vi "Dashboard Main.vi"() -> ()   [LabVIEW 2020]
uses:
  <vilib>/Utility/miscctls.llb/LVRectTypeDef.ctl
  <vilib>/event_ctls.llb/eventvkey.ctl
  <vilib>/Rock Robotics/WPI/DriverStation/WPI_DriverStationAllianceInfo.ctl
  b1c29fd4-b69e-4c47-bd92-218700034153.vi
  efc637a3-a7e0-4d6a-acb3-aee6468bd1cb.vi
  b2059994-562a-4507-8104-e4c00853bec9.vi
  7fc597ec-ac8e-4325-b133-71466b1fbbcb.vi
  9cac3b8b-4a3f-4d18-bfb1-3aae72e664f2.vi
  a7551b2b-ce58-4830-98e7-c5cf61f6feb4.vi
  cd51690b-7cbe-44fb-a5f0-3232adb0ed53.vi
  a4e8d5d1-2ec3-4e81-be0b-60391cc68073.vi
  1b78be80-bab2-445d-a3e8-82f142a16380.vi
  9e807339-2903-4f51-8fcc-64b6a9381567.vi
  e75f20ac-3dfa-4544-8614-4803d6d17fbb.vi
  273c17a0-a238-4f2a-a55a-7e29d73850ff.vi
  87bdd142-1820-4e26-8582-f713a5f3da40.vi
  b8451b18-7b16-4e07-a196-a1bebf8ce026.vi
  5d307e9f-edd0-4132-a387-09c5916d43b1.vi
  0137daef-9682-45ba-80b9-2d4fda8852b8.vi
  f6a63fab-964b-4051-8314-d4414a0a258c.vi
  90e0fe9d-42b1-4a72-a6c8-4b9d9b3a5a2a.vi
  f15e925d-3118-43e3-bf67-a1272bbf81dd.vi
  394886aa-4cdd-4740-8681-89e3e438764a.vi
  77a42c1f-99bf-4bb6-8218-45b49017f7dc.vi
  5abae45b-ab2b-4816-ba0c-2a0b218f6531.vi
  31f70c1d-3051-4c77-9544-a691198ba614.vi
  f63f5451-5db6-487e-bc86-5cb81e92b132.vi
  81d0db6a-d68a-45c3-b3b1-458879412541.vi
  c235c188-eb56-46fb-93d3-e8acf396af31.vi
  115ba94a-0b26-47fa-ae73-5ec5bd9e502a.vi
  2422668c-951b-48e5-9bda-0f59c56d9c0d.vi
  7776664e-4af7-4b3d-b288-2266642a045e.vi
  6004ed5d-dfc4-4dad-95c1-8e371ea2b9cd.vi
  321ce103-7778-4bb1-9ecc-75a76fef05e9.vi
  d30e88cc-5e2b-4867-b271-53fc6d5cd4d7.vi
  fde90579-e212-4b8a-8145-a17c3e40bcbd.vi
  6c63589b-432e-4f9c-bacb-2063ed7bd576.vi
  b7dcf304-99f6-4f78-9d14-19aa8d9ea562.vi
  e8b3bb93-ba91-445b-94c6-9e998421f827.vi
  0480a820-69ef-45e6-a9f4-d7ff60c89e45.vi
  1c99237e-ea3d-4ecf-b7c2-61034db3ecd2.vi
  0a8fe2ab-d060-4915-a9b5-d8978247e2b6.vi
  bcb69d65-de6b-4edb-ab22-bddb8ff6e42b.vi
  9102154a-bccf-464c-9607-78527809ea41.vi
  bef7421f-6b7f-4c9f-a030-6027c2463e15.vi
  88deb554-0c34-4998-a7e4-ba2d14003654.vi
  b1c29fd4-b69e-4c47-bd92-218700034153.vi/77c742ae-e671-49bb-a825-a6e8cebc9f63.vi
  b2059994-562a-4507-8104-e4c00853bec9.vi/77c742ae-e671-49bb-a825-a6e8cebc9f63.vi
  9cac3b8b-4a3f-4d18-bfb1-3aae72e664f2.vi/77c742ae-e671-49bb-a825-a6e8cebc9f63.vi
  a7551b2b-ce58-4830-98e7-c5cf61f6feb4.vi/77c742ae-e671-49bb-a825-a6e8cebc9f63.vi
  cd51690b-7cbe-44fb-a5f0-3232adb0ed53.vi/77c742ae-e671-49bb-a825-a6e8cebc9f63.vi
  a4e8d5d1-2ec3-4e81-be0b-60391cc68073.vi/77c742ae-e671-49bb-a825-a6e8cebc9f63.vi
  1b78be80-bab2-445d-a3e8-82f142a16380.vi/77c742ae-e671-49bb-a825-a6e8cebc9f63.vi
  9e807339-2903-4f51-8fcc-64b6a9381567.vi/77c742ae-e671-49bb-a825-a6e8cebc9f63.vi
  e75f20ac-3dfa-4544-8614-4803d6d17fbb.vi/77c742ae-e671-49bb-a825-a6e8cebc9f63.vi
  0137daef-9682-45ba-80b9-2d4fda8852b8.vi/77c742ae-e671-49bb-a825-a6e8cebc9f63.vi
  f6a63fab-964b-4051-8314-d4414a0a258c.vi/77c742ae-e671-49bb-a825-a6e8cebc9f63.vi
  90e0fe9d-42b1-4a72-a6c8-4b9d9b3a5a2a.vi/77c742ae-e671-49bb-a825-a6e8cebc9f63.vi
  f15e925d-3118-43e3-bf67-a1272bbf81dd.vi/77c742ae-e671-49bb-a825-a6e8cebc9f63.vi
  394886aa-4cdd-4740-8681-89e3e438764a.vi/77c742ae-e671-49bb-a825-a6e8cebc9f63.vi
  77a42c1f-99bf-4bb6-8218-45b49017f7dc.vi/77c742ae-e671-49bb-a825-a6e8cebc9f63.vi
  5abae45b-ab2b-4816-ba0c-2a0b218f6531.vi/77c742ae-e671-49bb-a825-a6e8cebc9f63.vi
  31f70c1d-3051-4c77-9544-a691198ba614.vi/77c742ae-e671-49bb-a825-a6e8cebc9f63.vi
  f63f5451-5db6-487e-bc86-5cb81e92b132.vi/77c742ae-e671-49bb-a825-a6e8cebc9f63.vi
  81d0db6a-d68a-45c3-b3b1-458879412541.vi/77c742ae-e671-49bb-a825-a6e8cebc9f63.vi
  c235c188-eb56-46fb-93d3-e8acf396af31.vi/77c742ae-e671-49bb-a825-a6e8cebc9f63.vi
  115ba94a-0b26-47fa-ae73-5ec5bd9e502a.vi/77c742ae-e671-49bb-a825-a6e8cebc9f63.vi
  2422668c-951b-48e5-9bda-0f59c56d9c0d.vi/77c742ae-e671-49bb-a825-a6e8cebc9f63.vi
  7776664e-4af7-4b3d-b288-2266642a045e.vi/77c742ae-e671-49bb-a825-a6e8cebc9f63.vi
  6004ed5d-dfc4-4dad-95c1-8e371ea2b9cd.vi/77c742ae-e671-49bb-a825-a6e8cebc9f63.vi
  321ce103-7778-4bb1-9ecc-75a76fef05e9.vi/77c742ae-e671-49bb-a825-a6e8cebc9f63.vi
  d30e88cc-5e2b-4867-b271-53fc6d5cd4d7.vi/77c742ae-e671-49bb-a825-a6e8cebc9f63.vi
  fde90579-e212-4b8a-8145-a17c3e40bcbd.vi/77c742ae-e671-49bb-a825-a6e8cebc9f63.vi
  6c63589b-432e-4f9c-bacb-2063ed7bd576.vi/77c742ae-e671-49bb-a825-a6e8cebc9f63.vi
  b7dcf304-99f6-4f78-9d14-19aa8d9ea562.vi/77c742ae-e671-49bb-a825-a6e8cebc9f63.vi
  e8b3bb93-ba91-445b-94c6-9e998421f827.vi/77c742ae-e671-49bb-a825-a6e8cebc9f63.vi
  0480a820-69ef-45e6-a9f4-d7ff60c89e45.vi/77c742ae-e671-49bb-a825-a6e8cebc9f63.vi
  1c99237e-ea3d-4ecf-b7c2-61034db3ecd2.vi/77c742ae-e671-49bb-a825-a6e8cebc9f63.vi
  0a8fe2ab-d060-4915-a9b5-d8978247e2b6.vi/77c742ae-e671-49bb-a825-a6e8cebc9f63.vi
  bcb69d65-de6b-4edb-ab22-bddb8ff6e42b.vi/77c742ae-e671-49bb-a825-a6e8cebc9f63.vi
  9102154a-bccf-464c-9607-78527809ea41.vi/77c742ae-e671-49bb-a825-a6e8cebc9f63.vi
  bef7421f-6b7f-4c9f-a030-6027c2463e15.vi/77c742ae-e671-49bb-a825-a6e8cebc9f63.vi
  88deb554-0c34-4998-a7e4-ba2d14003654.vi/77c742ae-e671-49bb-a825-a6e8cebc9f63.vi
  <vilib>/Utility/xml.llb/Read From XML File(array).vi
  <vilib>/Utility/xml.llb/Write to XML File(string).vi
  <vilib>/Rock Robotics/Network Tables/NT Read Number.vi
  <vilib>/Rock Robotics/Network Tables/NT Read Boolean.vi
  GlobalDashboard.vi
  <vilib>/Rock Robotics/Network Tables/NT Read String.vi
  <vilib>/Rock Robotics/Network Tables/NT Write Number.vi
  <vilib>/Rock Robotics/Network Tables/NT Read Numeric Array.vi
  <vilib>/Rock Robotics/Network Tables/NT Write Boolean.vi
  <vilib>/Rock Robotics/Network Tables/NT Read String Array.vi
  <vilib>/Rock Robotics/Network Tables/NT Write String.vi
  <vilib>/Rock Robotics/Network Tables/NT Write Numeric Array.vi
  <vilib>/Rock Robotics/Network Tables/NT Write Integer Array.vi
  <vilib>/Rock Robotics/Network Tables/NT Write Boolean Array.vi
  <vilib>/Rock Robotics/Network Tables/NT Write String Array.vi
  <vilib>/vision/NI_Vision_Development_Module.lvlib
panel:
  in  "TCP":refnum<k5>
  in  "Dashboard Tab":T1(tab)=enum."Setup/Auto"
  in  "CheckList":i32(listbox)
  out "TOF_Range":dbl format="%.1f"
  in  "Apply_Grid_Calibration":bool
  out "Current_Red_Calibration":dbl format="%.1f"
  in  "New_Red_Calibration":dbl format="%.1f"
  out "Heading_to_Target":dbl format="%.1f"
  out "Distance_to_Target":dbl format="%.1f"
  out "Robot_P":dbl format="%.1f"
  in  "Enable_Streaming_GUI":bool=TRUE
  out "Robot_Profile_GUI":string
  out "Auto_Playbook_GUI":string
  in  "Select Driver Profile":u16(ring) items=["N/A"]
  in  "Camera Name":string(combo)="limelight"
  in  "Camera Settings":T2={"Frame Rate"=20, "Compression"=60, "Size"=1, "DB Camera Config"=FALSE} {"Size" items=["640x480", "320x240", "160x120"]}
  in  "Select Autonomous Play":u16(ring) items=["N/A"]
  out "Master_Caution_GUI_0":bool caption="Mode_Butterfly"
  out "Robot_is_Autonomous_GUI_0":bool caption="Mode_Butterfly"
  out "Robot_Code_Version_GUI":string
  out "Auto_Suffix_GUI":string
  in  "Refresh_Auto_Play_List_GUI":bool
  in  "Auto_Delay_GUI":dbl format="%.1f"
  in  "Manual_Start_X":dbl min=0.0 max=700.0 format="%.1f"
  out "Robot_X":dbl format="%.1f"
  out "Robot_Y":dbl format="%.1f"
  in  "Manual_Start_Y":dbl min=0.0 max=400.0 format="%.1f"
  out "Robot_H_GUI":dbl format="%.1f"
  in  "Manual_Start_H":dbl min=0.0 max=360.0 format="%.1f"
  in  "Field Map":u16(ring) items=["N/A"]
  in  "Push_Robot_Start_GUI":bool
  in  "Export_Robot_Pose":bool
  in  "Clear_Robot_Pose_Display":bool
  in  "Dock_Dashboard":bool
  in  "Force_Human_Control_GUI":bool
  in  "Auto_Test_Mode_GUI":bool
  in  "Disable_Fusion_While_Autonomous":bool
  in  "Disable_Fusion_While_Disabled":bool=TRUE
  out "Robot Pose 1":cluster{dbl[], dbl[]}[](graph)
  in  "New_Blue_Calibration":dbl format="%.1f"
  out "Current_Blue_Calibration":dbl format="%.1f"
  out "Help Graphic":T3(plugin-control)
  out "LL_Ret_Left":bool
  out "LL_Ret_Right":bool
  out "WA_Ret_Right":bool
  out "WA_Ret_Left":bool
  out "Swerve_Drive_Fault":bool
  out "Robot Pose 2":cluster{dbl[], dbl[]}[](graph)
  out "Vision_Fault_GUI":bool
  out "Pressure_Leak_GUI":bool
  in  "Master_Safety_Override_1":bool
  in  "Manipulator_Help":bool
  in  "Driver_Help":bool
  out "No_Secondary_Camera":bool
  out "Swerve_Shifter_Failure":bool
  out "Electrical_Fault_GUI":bool
  out "Diverting_Power_GUI":bool
  out "CAN_Bus_Fault_GUI":bool
  out "IMU_Failure_GUI":bool
  out "Robot_is_Autonomous_GUI_1":bool caption="Mode_Butterfly"
  out "LL_Valid":bool caption="Mode_Butterfly"
  out "Auto_Error_GUI":bool
  in  "Clear_Errors_GUI":bool
  out "Swerve_Azimuth_Fault":bool
  out "Pressure_Transducer_GUI":dbl(slide) scale=0.0..115.0
  out "Pressure_Vent_GUI":bool
  out "Swerve_Overheating":bool
  out "Compressor_On_GUI":bool
  in  "Right":bool
  in  "Reticule":T4(ring)
  in  "Save":bool
  in  "Up":bool
  in  "Down":bool
  in  "Left":bool
  out "Master_Caution_GUI_1":bool caption="Mode_Butterfly"
  out "Battery_Critical_GUI":bool
  out "Battery_Voltage_GUI":dbl(slide) scale=11.0..13.0
  out "Field_Oriented_GUI":bool caption="Mode_Butterfly"
  out "Slow_Loop":bool
  out "Combined Camera Feed":T3(plugin-control)
  in  "Camera_Override_GUI":bool
  in  "Field_Oriented_Override_GUI":bool
  out "Pointed_at_Target":bool caption="Mode_Butterfly"
  in  "Auto_Targeting_Override":bool
  out "Using_Auto_Targeting":bool caption="Mode_Butterfly"
  out "Solenoid 4 Numeric Display":dbl
  out "Sensor 4 Boolean Display":bool
  out "Solenoid 3 Numeric Display":dbl
  out "Sensor 3 Boolean Display":bool
  out "Solenoid 2 Numeric Display":dbl
  out "Sensor 2 Boolean Display":bool
  out "Solenoid 1 Numeric Display":dbl
  out "Sensor 1 Boolean Display":bool
  in  "Motor 8 Button Selector":T5(ring)
  in  "Motor 8 Amplitude":dbl(slide) caption="Slide" min=-1.0 max=1.0 step=0.1 scale=-1.0..1.0
  in  "Motor 7 Button Selector":T5(ring)
  in  "Motor 7 Amplitude":dbl(slide) caption="Slide" min=-1.0 max=1.0 step=0.1 scale=-1.0..1.0
  in  "Motor 6 Button Selector":T5(ring)
  in  "Motor 6 Amplitude":dbl(slide) caption="Slide" min=-1.0 max=1.0 step=0.1 scale=-1.0..1.0
  in  "Motor 5 Button Selector":T5(ring)
  in  "Motor 5 Amplitude":dbl(slide) caption="Slide" min=-1.0 max=1.0 step=0.1 scale=-1.0..1.0
  in  "Motor 4 Button Selector":T5(ring)
  in  "Motor 4 Amplitude":dbl(slide) caption="Slide" min=-1.0 max=1.0 step=0.1 scale=-1.0..1.0
  in  "Motor 3 Button Selector":T5(ring)
  in  "Motor 3 Amplitude":dbl(slide) caption="Slide" min=-1.0 max=1.0 step=0.1 scale=-1.0..1.0
  in  "Motor 2 Button Selector":T5(ring)
  in  "Motor 2 Amplitude":dbl(slide) caption="Slide" min=-1.0 max=1.0 step=0.1 scale=-1.0..1.0
  in  "Solenoid 4 Toggle":bool
  in  "Solenoid 4 Selector":T6(ring)
  in  "Solenoid 3 Toggle":bool
  in  "Solenoid 3 Selector":T6(ring)
  in  "Solenoid 2 Toggle":bool
  in  "Solenoid 2 Selector":T6(ring)
  in  "Solenoid 1 Toggle":bool
  in  "Solenoid 1 Selector":T6(ring)
  in  "Motor 1 Button Selector":T5(ring)
  in  "Motor 1 Amplitude":dbl(slide) caption="Slide" min=-1.0 max=1.0 step=0.1 scale=-1.0..1.0
  out "Swerve_Output_Loop_Time_GU":u32
  out "Swerve_3_Drive_Velocity":dbl format="%.1f"
  out "Swerve_3_Azimuth_Position":dbl format="%.1f"
  out "Swerve_3_Drive_Temperature":dbl
  out "Swerve_0_Drive_Temperature":dbl
  out "Camera Perf":string
  out "Control_Loop_Time_GUI":u32
  in  "Calibrate_Wheels_GUI":bool
  in  "Home_Wheels_GUI":bool
  out "Swerve_0_Azimuth_Position":dbl format="%.1f"
  out "Swerve_0_Drive_Velocity":dbl format="%.1f"
  out "Swerve_1_Drive_Velocity":dbl format="%.1f"
  out "Swerve_1_Azimuth_Position":dbl format="%.1f"
  out "Swerve_1_Drive_Temperature":dbl
  out "Swerve_2_Drive_Velocity":dbl format="%.1f"
  out "Swerve_2_Azimuth_Position":dbl format="%.1f"
  out "Swerve_2_Drive_Temperature":dbl
  in  "Arm_Calibrate_Wheels_GUI":bool
  out "Master_Caution_GUI_2":bool caption="Mode_Butterfly"
  in  "Actuator Testing":u16(ring) items=["N/A"]
  in  "Test_Actuator_Value_GUI":dbl step=0.1 format="%.2f"
  in  "Calibrate_Joysticks_GUI":bool
  in  "Arm_Calibrate_Joysticks":bool
  out "Robot_is_Autonomous_GUI_2":bool caption="Mode_Butterfly"
  in  "Test_Actuator_Period_GUI":dbl min=0.0 step=1.0 format="%.2f"
  out "Pose_Loop_Time_GUI":u32
  in  "Mute_Audible_Warnings":bool
  out "Combined Error String":string
  out "Swerve_0_Shifter_State":string
  out "Swerve_1_Shifter_State":string
  out "Swerve_3_Shifter_State":string
  out "Swerve_2_Shifter_State":string
  out "Swerve_Azimuth_Fault_Array":bool[](array[boolean])
  in  "Super_Test_Mode_GUI":bool
  out "Current_Driver_Profile_Setpoints_GUI":T7={"Strafe Deadband"=0.08, "Strafe Scaling"=2.0, "Strafe Maximum"=0.5, "Rotation Deadband"=0.15, "Rotation Scaling"=2.5, "Rotation Maximum"=0.5} {"Rotation Maximum" min=0.3 max=1.0 scale=0.3..1.0; "Rotation Scaling" min=1.0 max=4.0 scale=1.0..4.0; "Rotation Deadband" min=0.0 max=0.25 scale=0.0..0.25; "Strafe Maximum" min=0.3 max=1.0 scale=0.3..1.0; "Strafe Scaling" min=1.0 max=4.0 scale=1.0..4.0; "Strafe Deadband" min=0.0 max=0.25 scale=0.0..0.25}
  in  "New_Driver_Profile_Setpoints_GUI":T8={"Strafe Deadband"=0.08, "Strafe Scaling"=2.0, "Strafe Max"=0.5, "Rotate Deadband"=0.15, "Rotate Scaling"=2.5, "Rotate Max"=0.5} {"Rotate Max" min=0.3 max=1.0 format="%.2g"; "Rotate Scaling" min=1.0 max=4.0 format="%.2g"; "Rotate Deadband" min=0.0 max=0.25 format="%.2g"; "Strafe Max" min=0.3 max=1.0 format="%.2g"; "Strafe Scaling" min=1.0 max=4.0 format="%.2g"; "Strafe Deadband" min=0.0 max=0.25 format="%.2g"}
  in  "Apply_Driver_Profile_Setpoints_GUI":bool
  out "Current_Driver_Profile_GUI":string
  in  "Free_Tuning_Variable_GUI":dbl min=0.0 step=1.0 format="%.3f"
  out "Audible_Warnings_Enabled_GUI":bool
  out "Legal_Drivers_GUI":string[](array[string])
  out "Swerve_Shifter_Failure_Array":bool[](array[boolean])
  out "Swerve_Overheating_Array":bool[](array[boolean])
  out "Swerve_Drive_Fault_Array":bool[](array[boolean])
  out "NT Connection":bool
  out "Mode":T9(ring)=enum."Auto Disabled"
  out "Tree":string(tree)
  out "Background":bool
  # "2023 Dashboard v2.3-stable"
  # "Robot Profile"
  # "Robot X Position (in)"
  # "Robot Y Position (in)"
  # "Delay (s)"
  # "Robot Heading (deg)"
  # "Suffix"
  # "X (in)"
  # "Robot Pitch (deg)"
  # "Autonomous Playbook Entry"
  # "Auto Test\nMode"
  # "Force\nHuman"
  # "Y (in)"
  # "Target Distance (in)"
  # "Target Heading (deg)"
  # "H (deg)"
  # "Hybrid Node  Sensor (in)"
  # "Undock Dashboard"
  # "Yes Camera Streaming"
  # "Stop Fusion While Auto"
  # "Stop Fusion While Disabled"
  # "Grid Y Calibration (in)"
  # "X"
  # "Y"
  # "MASTER\nSTATES"
  # "OVERRIDES"
  # "Camera Override"
  # "Robot-Oriented Drive Controls"
  # "Auto-Targeting Override"
  # "Disengage\nSafeties"
  # "11"
  # "13"
  # "0"
  # "120"
  # "Amplitude"
  # "Button"
  # "Button"
  # "Drivebase Subsytem"
  # "Driver Profile Selected"
  # "Loop Times"
  # "Module 1"
  # "Module 0"
  # "Motor 1"
  # "Solenoid 1"
  # "Control (ms)"
  # "Azimuth (deg)"
  # "Pose (ms)"
  # "Temp (C)"
  # "Motor 2"
  # "Solenoid 2"
  # "Drive Output (ms)"
  # "Velocity (ft/s)"
  # "Shifter State"
  # "Motor 3"
  # "Solenoid 3"
  # "Module 2"
  # "Module 3"
  # "Solenoid 4"
  # "Motor 4"
  # "Variable (bleh)"
  # "Disabled\nTest Mode"
  # "Azimuth (deg)"
  # "Temp (C)"
  # "Motor 5"
  # "Sensor 1"
  # "Velocity (ft/s)"
  # "Shifter State"
  # "Motor 6"
  # "Sensor 2"
  # "Calibrate Wheels"
  # "Motor 7"
  # "Sensor 3"
  # "Period (s)"
  # "Calibrate Joysticks"
  # "Amplitude"
  # "Motor 8"
  # "Sensor 4"
  # "0"
  # "0.25"
  # "1"
  # "4"
  # "0.3"
  # "1"
  # "0"
  # "0.25"
  # "1"
  # "4"
  # "0.3"
  # "1"
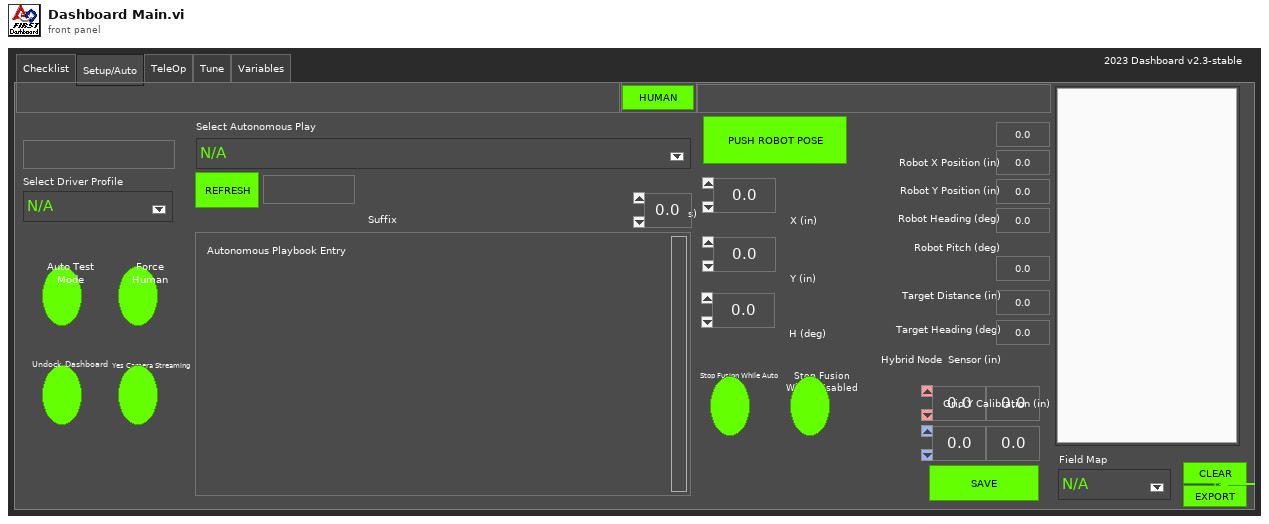
[diagram p1: front panel]
types:
  T1 = enum32{"Checklist", "Setup/Auto", "TeleOp", "Tune", "NT", "Test", "Commands", "Variables"}
  T2 = cluster{"Frame Rate":i32, "Compression":i32, "Size":u16, "DB Camera Config":bool}
  T3 = typedef "IMAQ Image.ctl" = refnum<image>
  T4 = enum16{"Wide Angle Left Reticule", "Wide Angle Right Reticule", "Lime Light Left Reticule", "Lime Light Right Reticule"}
  T5 = enum16{"Off", "Slider", "D_LT", "D_RT", "D_LB", "D_RB", "D_Y", "D_X", "D_A", "D_B", "M_LJoystick_X", "M_LJoystick_Y", "M_RJoystick_X", "M_RJoystick_Y", "M_LT", "M_RT", "M_LB", "M_RB", "M_Y", "M_X", "M_A", "M_B"}
  T6 = enum16{"Off", "Toggle", "D_LT", "D_RT", "D_LB", "D_RB", "D_Y", "D_X", "D_A", "D_B", "M_LT", "M_RT", "M_LB", "M_RB", "M_Y", "M_X", "M_A", "M_B"}
  T7 = cluster{"Strafe Deadband":dbl, "Strafe Scaling":dbl, "Strafe Maximum":dbl, "Rotation Deadband":dbl, "Rotation Scaling":dbl, "Rotation Maximum":dbl}
  T8 = cluster{"Strafe Deadband":dbl, "Strafe Scaling":dbl, "Strafe Max":dbl, "Rotate Deadband":dbl, "Rotate Scaling":dbl, "Rotate Max":dbl}
  T9 = enum8{"Tele-Op Disabled", "Tele-Op Enabled", "Auto Disabled", "Auto Enabled", "Test Disabled", "Test Enabled", "Disconnected", "No Code", "E-Stop"}
  T10 = cluster{"Save Path":path, "Interval (s)":dbl, "Keep":i32}
  T11 = enum32{"Drive", "Camera", "Basic", "Custom", "Test", "Commands", "Checklist", "Variables"}
  T12 = cluster{"IDs":cluster{"RPC field ID":u16, "Unique ID":u16}, "String":string}
  T13 = typedef "Image Type" = u32
  T14 = typedef "WPI_DriverStationAllianceInfo.ctl" = enum16{"Red", "Blue", "Invalid"}
  T15 = enum8{"Enabled", "Disabled", "Disabled and Grayed Out"}
  T16 = cluster{"Error Strings":string, "Disable Counts":cluster{u16, u16}, "Rail Faults":cluster{u16, u16, u16}, "Robot IP":string, "DB Mode":u8, "Event Info":cluster{"Name":string, "Type":u8, "Number":u16, "Replay":u8}}
  T17 = cluster{"Storage":cluster{"Disk Free":u64, "RAM Block":u32, "RAM free":u32}, "CPU Utilization":cluster{"CPU % ISR":sgl, "CPU % Time Crit":sgl, "CPU % Timed Str":sgl, "CPU % High":sgl, "CPU % Above":sgl, "CPU % Normal":sgl, "CPU % Low":sgl}, "CAN":cluster{"% Bus Utilization":sgl, "Bus Off Cnt":u32, "TX_FIFO Full Cnt":u32, "Receive Error Cnt":u8, "Transmit Error Cnt":u8}, "HID":cluster{"HID Outputs":u32, "Rumble Low":u16, "Rumble High":u16}[]}
  T18 = cluster{"Status bits":cluster{"Test Mode":bool, "Autonomous":bool, "Enabled":bool, "Code Start":bool, "Brownout":bool, "Reserved 2":bool, "Reserved 3":bool, "E-Stop":bool}, "Code Trace":cluster{"Disabled":bool, "TeleOp":bool, "Auto":bool, "Test":bool}, "Controller Type":enum16{"unknown", "cRIO", "roboRio"}, "Code?":enum16{"unknown", "noCode", "code"}, "Battery V":dbl}
  T19 = cluster{"Control Bits":cluster{"TestMode":bool, "Autonomous":bool, "Enabled":bool, "FMS Present":bool, bool, bool, bool, "E-Stop":bool}, "Team Station ":u8, "Countdown":sgl, "Joystick Values":cluster{"Axes":dbl[], "Buttons":bool[], "POVs":i16[]}[]}
  T20 = typedef "imagedata.ctl" = cluster{"image type":i32, "image depth":i32, "image":u8[], "mask":u8[], "colors":u32[], "Rectangle":cluster{"left":i16, "top":i16, "right":i16, "bottom":i16}}
  T21 = cluster{"Boolean":bool, "Numeric Text.Text Colors:Text Color":u32}
  T22 = cluster{"value[0]":dbl, "value[1]":dbl, "value[2]":dbl, "value[3]":dbl, "value[4]":dbl, "value[5]":dbl}
  T23 = enum16{"Off", "Toggle", "D_LT", "D_RT", "D_LB", "D_RB", "D_Y", "D_X", "D_A", "D_B", "M_LT", "M_RT", "M_LB", "M_RB", "M_Y", "M_X", "M_A", "M_B"}[]
  T24 = enum16{"Off", "Slider", "D_LT", "D_RT", "D_LB", "D_RB", "D_Y", "D_X", "D_A", "D_B", "M_LJoystick_X", "M_LJoystick_Y", "M_RJoystick_X", "M_RJoystick_Y", "M_LT", "M_RT", "M_LB", "M_RB", "M_Y", "M_X", "M_A", "M_B"}[]
  T25 = typedef "LVRectTypeDef.ctl" = cluster{"Left":i16, "Top":i16, "Right":i16, "Bottom":i16}
  T26 = typedef "eventvkey.ctl" = enum16{"ASCII", "Enter", "Return", "Shift", "Ctrl", "Alt", "Cmd", "Opt", "Caps", "NumLock", "Clear", "Break", "Up", "Down", "Left", "Right", "Insert", "Delete", "Home", "End", "PageUp", "PageDown", "Escape", "Help", "Pause", "ScrollLock", "F1", "F2", "F3", "F4", "F5", "F6", "F7", "F8", "F9", "F10", "F11", "F12", "F13", "F14", "F15", "F16", "F17", "F18", "F19", "F20", "F21", "F22", "F23", "F24", "Play", "VolumeUp", "VolumeDown", "Mute", "Two Byte Char"}
  T27 = cluster{"Shift":bool, "Ctrl":bool, "Alt":bool, "Cmd":bool, "Opt":bool}
  T28 = cluster{"WA_Ret_Left":refnum<vi>, "WA_Ret_Right":refnum<vi>, "LL_Ret_Left":refnum<vi>, "LL_Ret_Right":refnum<vi>}
  T29 = cluster{"Camera Name":string, string, "Saved DB Images Info":cluster{"Save Path":path, "Interval (s)":dbl, "Keep":i32}}
  T30 = cluster{string, "Swerve_Shifter_Failure":bool, dbl}
  T31 = cluster{string, "Master_Safety_Override_1":bool, dbl}
  T32 = cluster{string, "Swerve_Azimuth_Fault":bool, dbl}
  T33 = cluster{string, "Arm_Calibrate_Wheels_GUI":bool, dbl}
  T34 = cluster{string, "Electrical_Fault_GUI":bool, dbl}
  T35 = cluster{string, "Arm_Calibrate_Joysticks":bool, dbl}
  T36 = cluster{string, "Swerve_Drive_Fault":bool, dbl}[]
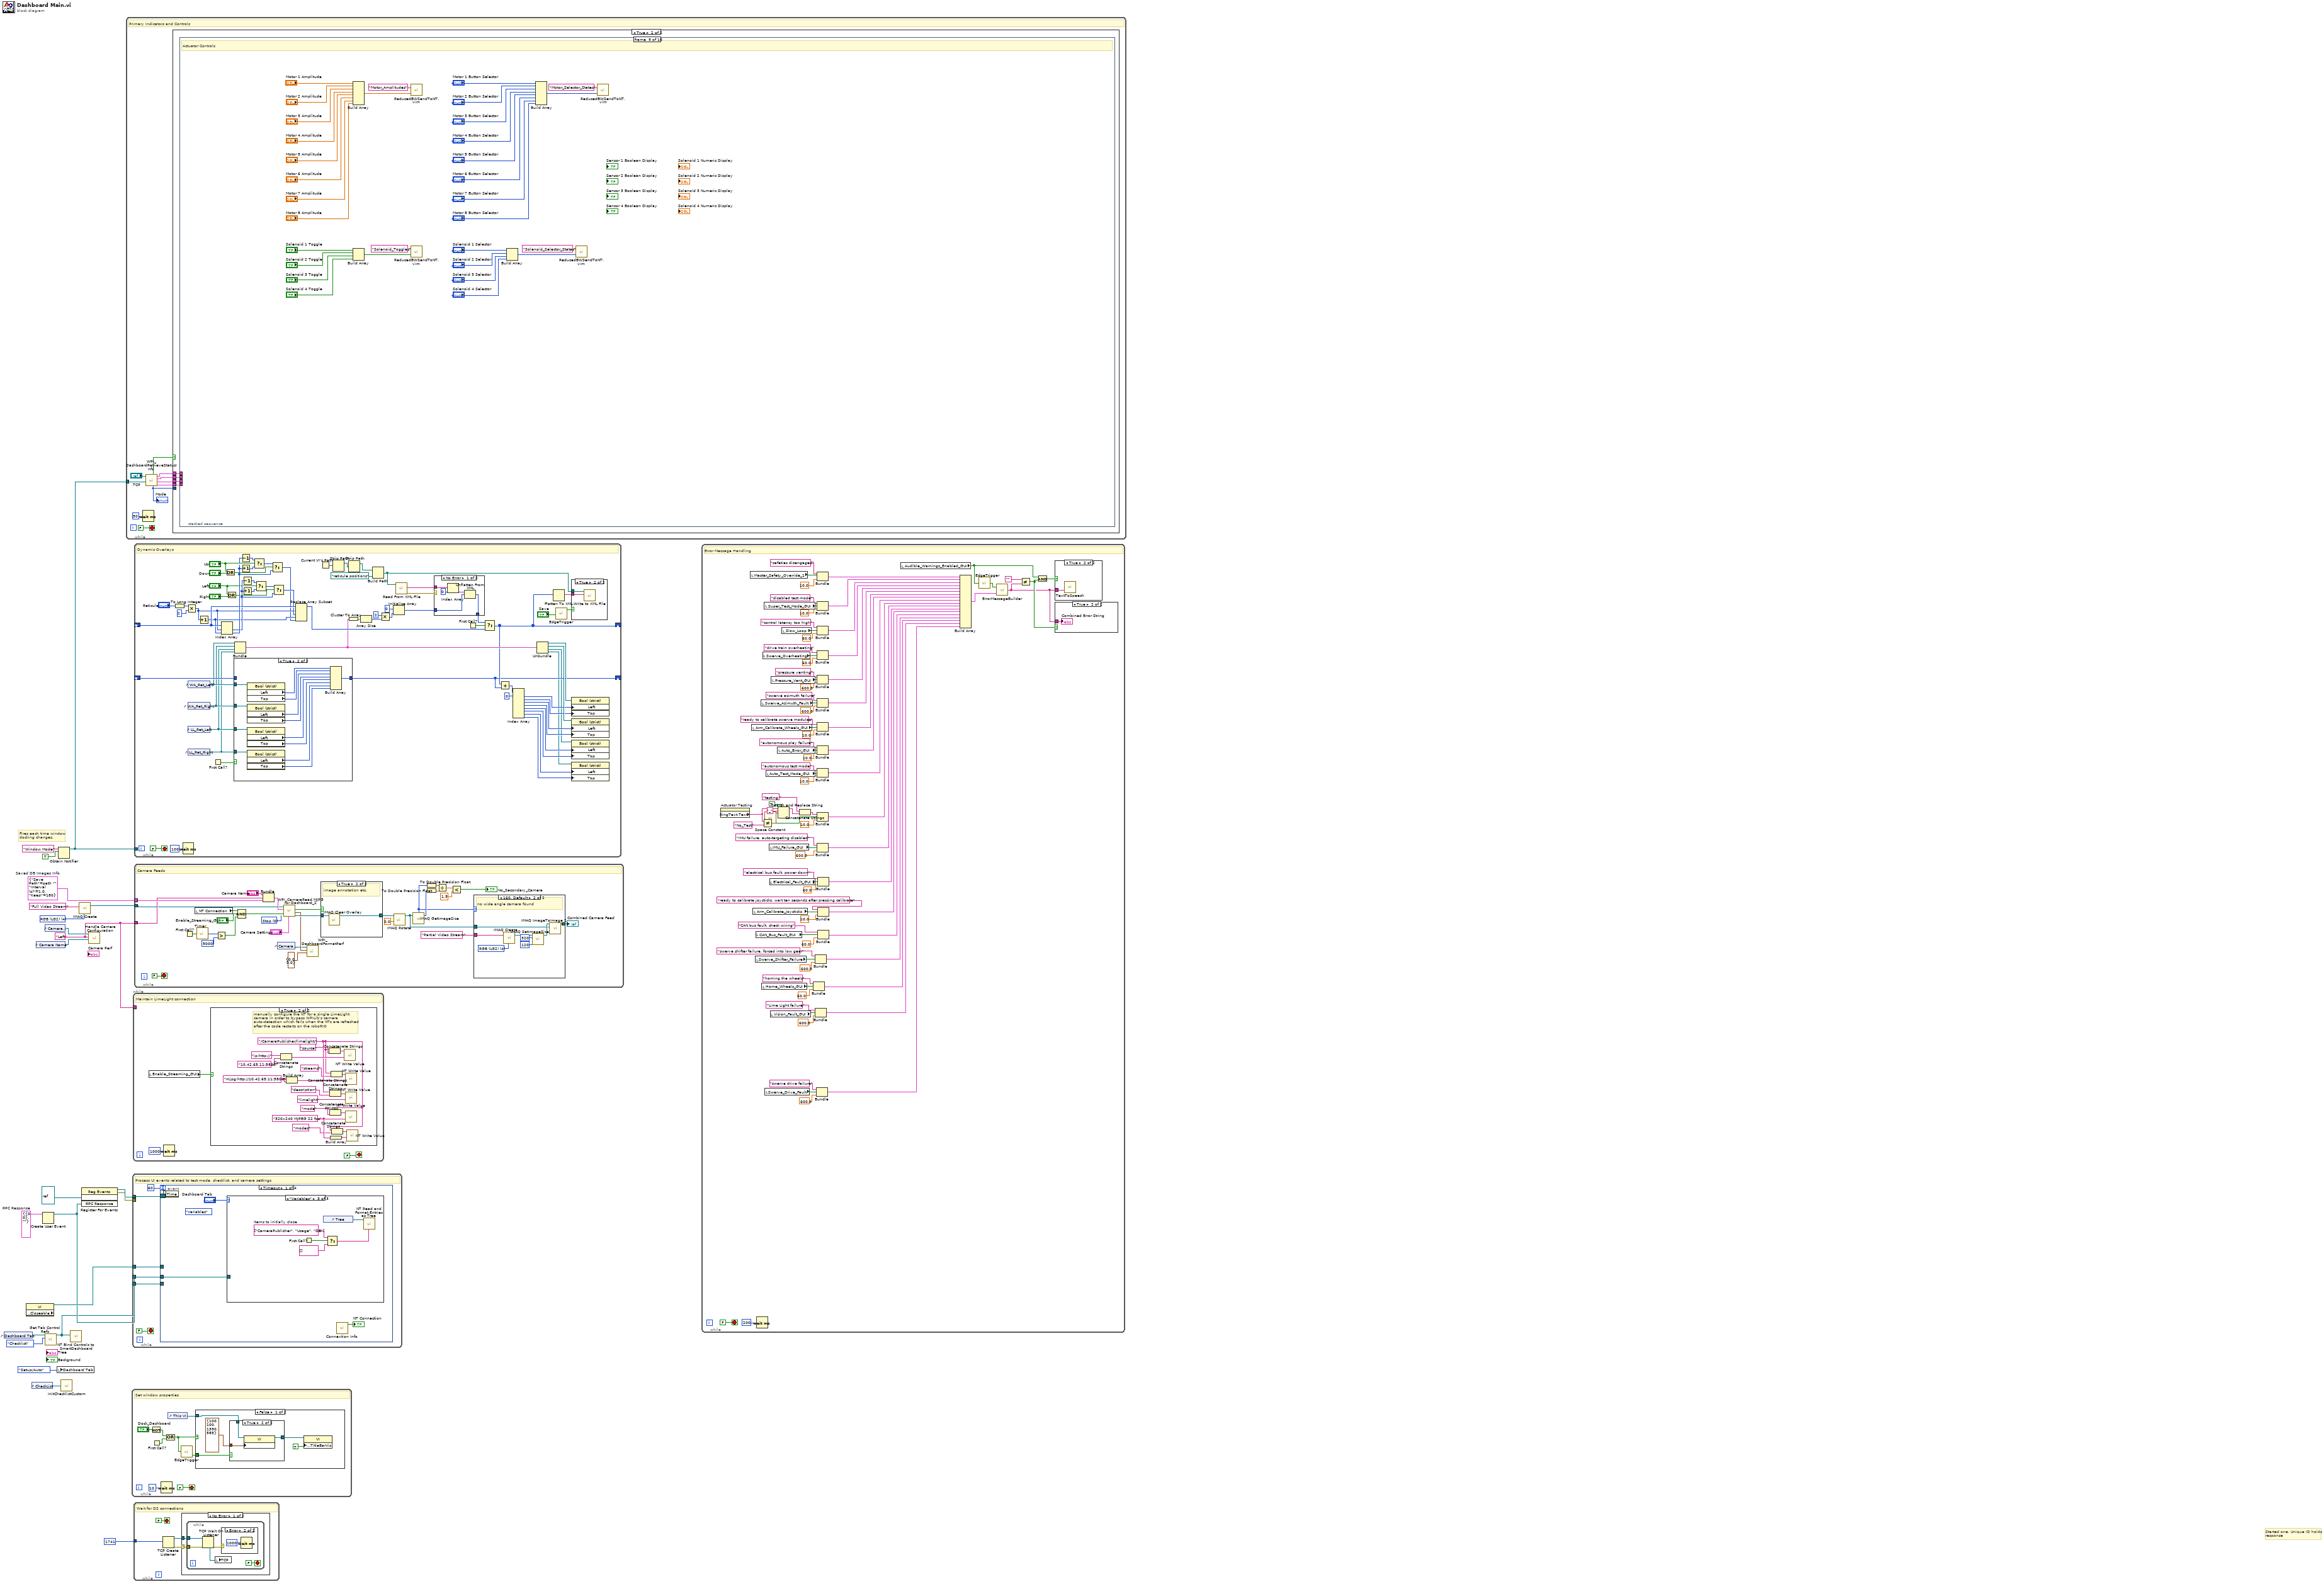
[diagram p0: block diagram]
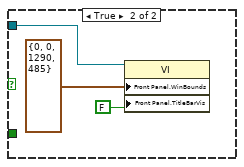
[diagram p4: hidden frame]
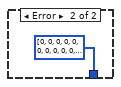
[diagram p7: hidden frame]
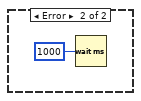
[diagram p11: hidden frame]
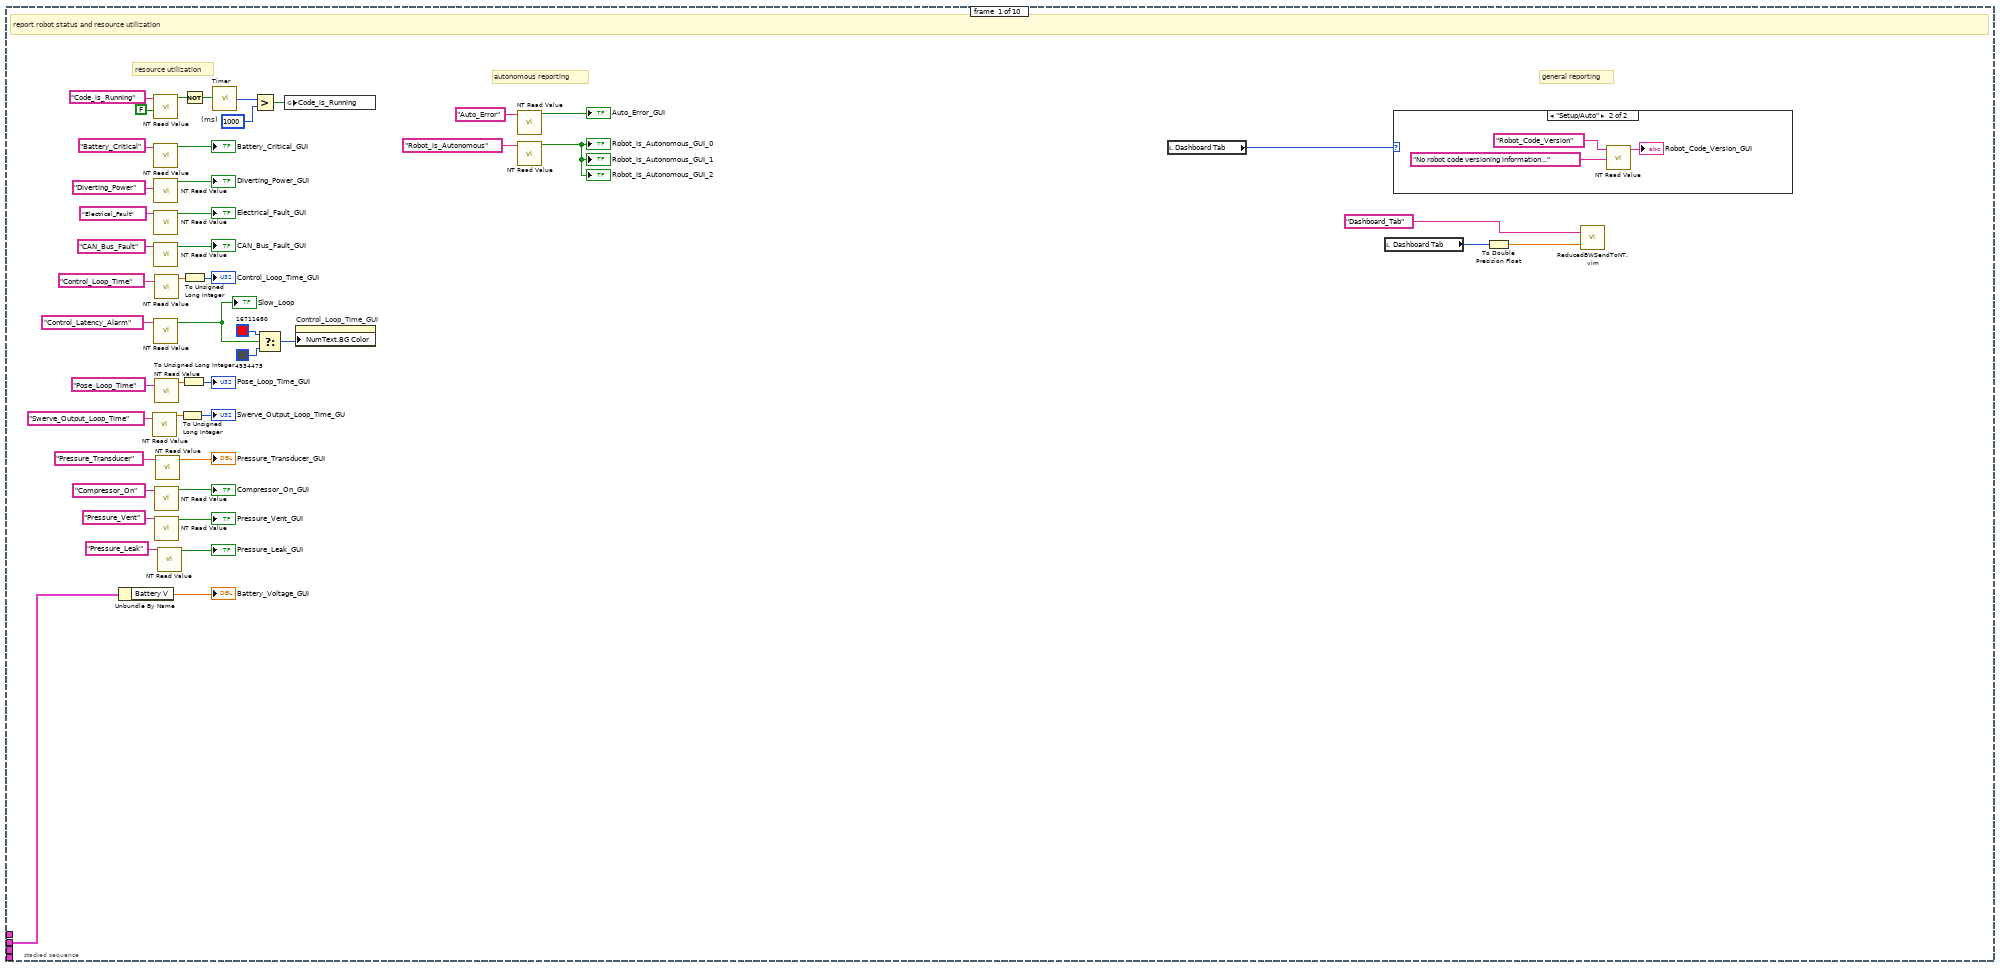
[diagram p13: hidden frame]
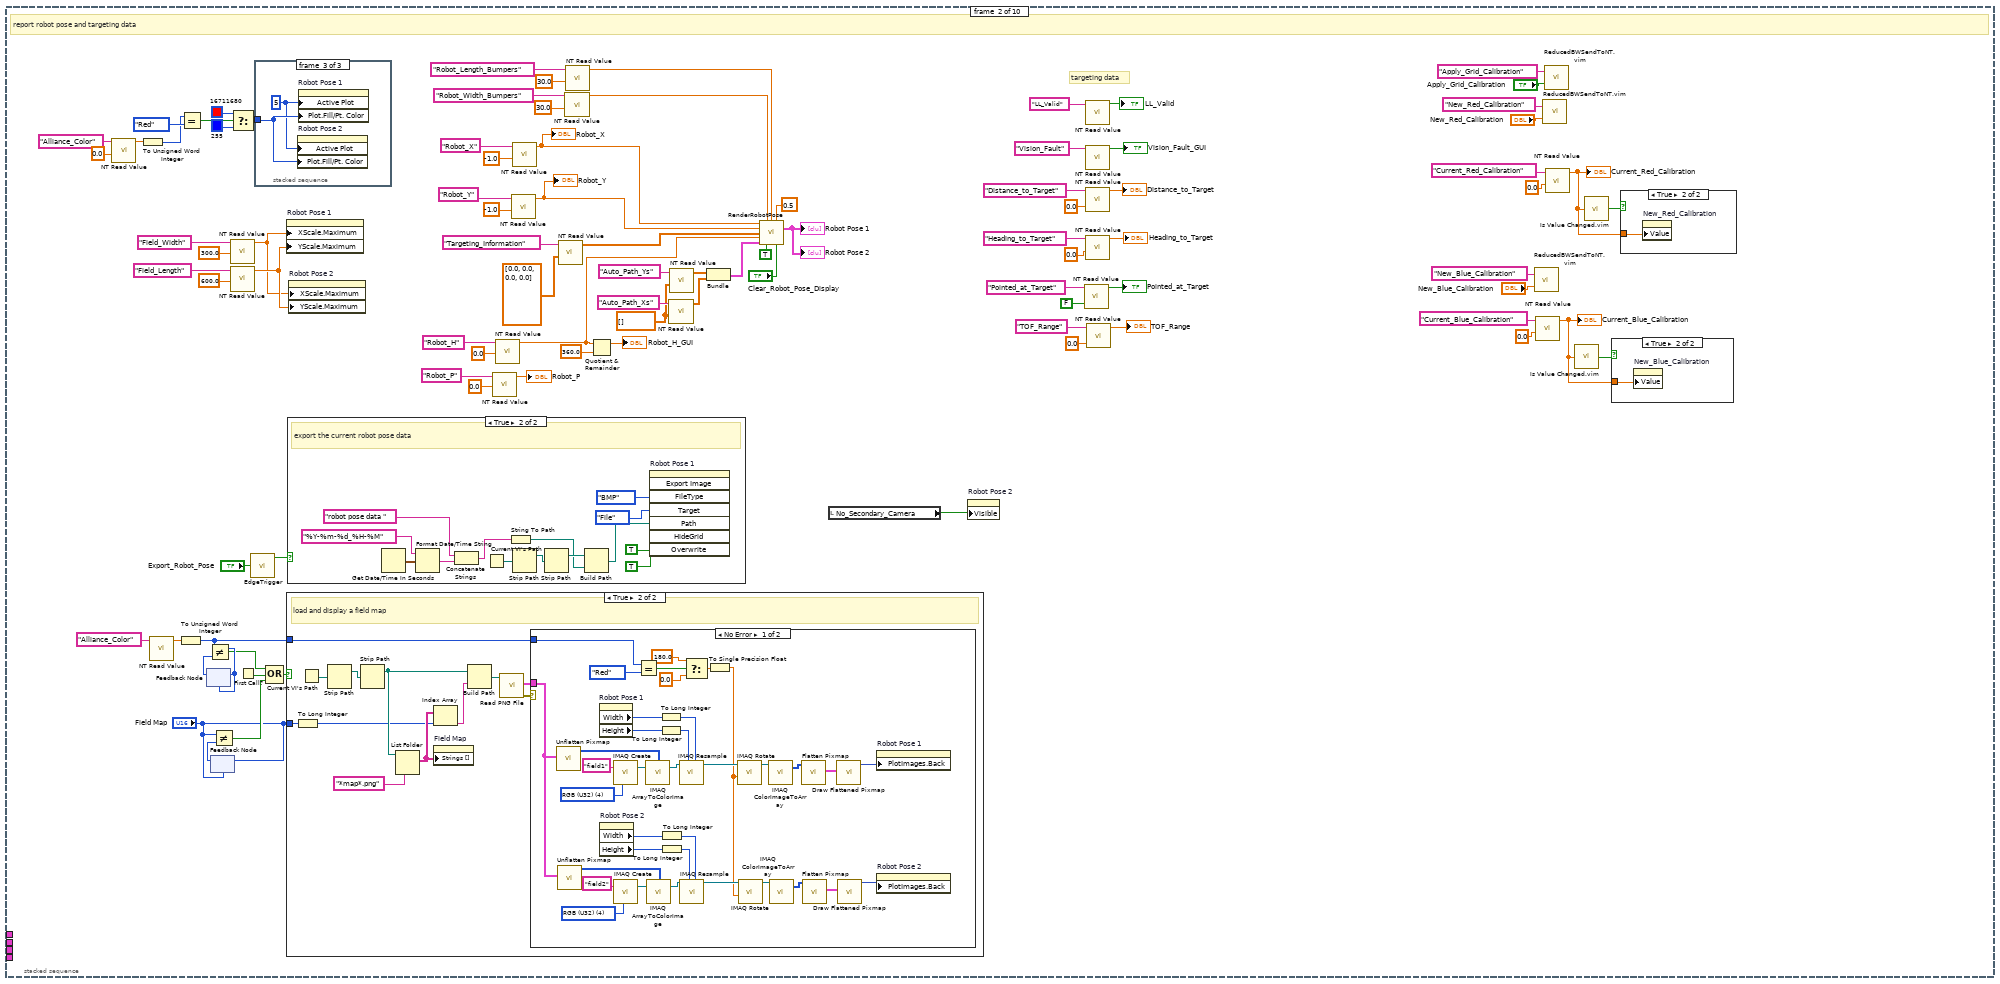
[diagram p15: hidden frame]
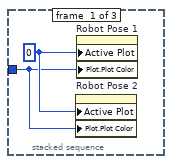
[diagram p18: hidden frame]
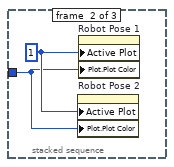
[diagram p19: hidden frame]
diagram:
  w10 = T10 {"Save Path"=path "", "Interval (s)"=1.0, "Keep"=180}  # Saved DB Images Info
  w3 = "Left"
  w13 = T12 {"IDs"={"RPC field ID"=0, "Unique ID"=0}, "String"=""}  # RPC Response
  w6 = T13 4 items=["Grayscale (U8)", "Grayscale (I16)", "Grayscale (SGL)", "Complex (CSG)", "RGB (U32)", "HSL (U32)", "RGB (U64)"] ("Image Type")
  # "Started one, Unique ID holds\nresponse"
  # "Fires each time window\ndocking changes."
  n1 = control-ref of="Dashboard Tab"() -> (w16:refnum<vi>)
  n2 = property class="VI" props=["Front Panel.Closeable"]() -> (reference out=w17:refnum<vi>)  [unwired: 2 in, 2 out]
  n3 = control-ref of="CheckList"() -> (w5:refnum<vi>)
  n4 = control-ref of="Camera Name"() -> (w8:refnum<vi>)
  n5 = Create User Event(user event datatype=w13) -> (user event=w12:refnum<user-event>)  [unwired: 1 in, 1 out]
  n6 = control-ref of="Camera Settings"() -> (w9:refnum<vi>)
  n7 = call <vilib>:"Get Tab Control Refs.vi"("Page Index"=T11."Checklist" ("Dashboard Tab"), "TabControl in"=w16) -> ("ControlsOnPage"=w2:refnum<vi>[])  [unwired: 9 in]
  n8 = local write "Dashboard Tab"(T1."Setup/Auto" ("Dashboard Tab")) -> ()
  n9 = Obtain Notifier(name (unnamed)="Window Mode", notification data type=TRUE) -> (notifier out=w1:refnum<notifier>)  [unwired: 2 in, 2 out]
  n10 = call "InitChecklistCustom.vi"("ListBox in"=w5) -> ()  [unwired: 1 in]
  n11 = call <vilib>:"NT Bind Controls to SmartDashboard.vi"("Bound Control Refs"=w2) -> ()  [unwired: 11 in]
  n12 = call "IMAQ Create"("Image Name"="Full Video Stream", "Image Type"=w6) -> ("New Image"=w4:T3)  [unwired: 2 in, 2 out]
  n13 = register-events(refnum<vi> refnum, w12) -> (reference out=w20:refnum<event-registration>, error out=w19:errorcluster)  [unwired: 2 in]
  n14 = call "Handle Camera Configuration.vi"("CameraNameRef"=w8, "Display Name"=w3, "ClusterRef"=w9) -> ()  [unwired: 9 in]
  n15 = while {
    tunnel: w1 -> [w24]
    stop <- FALSE stop-if-true
    # "Primary Indicators and Controls"
    n16 = Wait (ms)(milliseconds to wait=u32 50) -> ()  [unwired: 1 out]
    n17 = call <vilib>:"WPI_DashboardRetrieveStatusInfo.vi"("Window Mode Notifier"=w24, "TCP Cnx"="TCP") -> ("Power and Errors"=w27:T16, "Robot Metrics"=w30:T17, "Status Info"=w31:T18, "Control Info"=w28:T19, "Robot Mode"=w26:T9, "Process?"=w29:bool)  [unwired: 4 in]
    "Mode" <- w26
    n18 = case shown="True" w29 {
      tunnel: w31 -> [_ w35]
      tunnel: w30 -> [_ w34]
      tunnel: w28 -> [_ w36]
      tunnel: w27 -> [_ w33]
      tunnel: w26 -> [_ _]
      frame False {
      }
      frame True {
        n19 = stacked-sequence {
          tunnel: w36 -> [_ _ _ _ _ _ _ _ _ _]
          tunnel: w35 -> [w51 _ _ _ _ _ _ _ _ _]
          tunnel: w34 -> [_ _ _ _ _ _ _ _ _ _]
          tunnel: w33 -> [_ _ _ _ _ _ _ _ _ _]
          frame #0 {
            w41 = u32 1000  # (ms)
            # "general reporting"
            # "resource utilization"
            # "autonomous reporting"
            # "report robot status and resource utilization"
            n20 = Unbundle By Name(w51) -> ("Battery V"=→"Battery_Voltage_GUI":dbl)
            n21 = call-poly <vilib>:"NT Read Value.vi"("name"="Swerve_Output_Loop_Time" ("Name")) -> ("value"=w39:dbl)  [unwired: 8 in, 2 out]
            n22 = call-poly <vilib>:"NT Read Value.vi"("default value"=FALSE, "name"="Code_is_Running" ("Name")) -> ("value"=w44:bool)  [unwired: 7 in, 2 out]
            n23 = call-poly <vilib>:"NT Read Value.vi"("name"="Battery_Critical" ("Name")) -> ("value"=→"Battery_Critical_GUI":bool)  [unwired: 8 in, 2 out]
            n24 = call-poly <vilib>:"NT Read Value.vi"("name"="Diverting_Power" ("Name")) -> ("value"=→"Diverting_Power_GUI":bool)  [unwired: 8 in, 2 out]
            n25 = call-poly <vilib>:"NT Read Value.vi"("name"="Electrical_Fault" ("Name")) -> ("value"=→"Electrical_Fault_GUI":bool)  [unwired: 8 in, 2 out]
            n26 = call-poly <vilib>:"NT Read Value.vi"("name"="CAN_Bus_Fault" ("Name")) -> ("value"=→"CAN_Bus_Fault_GUI":bool)  [unwired: 8 in, 2 out]
            n27 = call-poly <vilib>:"NT Read Value.vi"("name"="Control_Latency_Alarm" ("Name")) -> ("value"=w80:bool)  [unwired: 8 in, 2 out]
            "Slow_Loop" <- w80
            n28 = call-poly <vilib>:"NT Read Value.vi"("name"="Control_Loop_Time" ("Name")) -> ("value"=w71:dbl)  [unwired: 8 in, 2 out]
            n29 = call-poly <vilib>:"NT Read Value.vi"("name"="Pose_Loop_Time" ("Name")) -> ("value"=w81:dbl)  [unwired: 8 in, 2 out]
            n30 = call-poly <vilib>:"NT Read Value.vi"("name"="Compressor_On" ("Name")) -> ("value"=→"Compressor_On_GUI":bool)  [unwired: 8 in, 2 out]
            n31 = call-poly <vilib>:"NT Read Value.vi"("name"="Pressure_Vent" ("Name")) -> ("value"=→"Pressure_Vent_GUI":bool)  [unwired: 8 in, 2 out]
            n32 = call-poly <vilib>:"NT Read Value.vi"("name"="Pressure_Transducer" ("Name")) -> ("value"=→"Pressure_Transducer_GUI":dbl)  [unwired: 8 in, 2 out]
            n33 = call-poly <vilib>:"NT Read Value.vi"("name"="Pressure_Leak" ("Name")) -> ("value"=→"Pressure_Leak_GUI":bool)  [unwired: 8 in, 2 out]
            n34 = To Unsigned Long Integer(number=w39) -> (unsigned 32bit integer=→"Swerve_Output_Loop_Time_GU":u32)
            n35 = To Unsigned Long Integer(number=w81) -> (unsigned 32bit integer=→"Pose_Loop_Time_GUI":u32)
            n36 = Not(x=w44) -> (.not. x?=w43:bool)
            n37 = To Unsigned Long Integer(number=w71) -> (unsigned 32bit integer=→"Control_Loop_Time_GUI":u32)
            n38 = call "Timer.vi"("Reset Timer"=w43) -> ("Time (ms)"=w42:u32)
            n39 = Greater?(x=w42, y=w41) -> (0:w40:bool)
            n40 = Select(t=u32 16711680 ("Numeric Text.Text Colors:Text Color"), s=w80, f=u32 4934475 ("Numeric Text.Text Colors:Text Color")) -> (s? t:f=w75:u32)
            n41 = global write "GlobalDashboard.vi" "Code_is_Running"(w40) -> ()
            n42 = property on="Control_Loop_Time_GUI" class="DigNum (strict)"("NumText.BG Color"=w75) -> ()  [unwired: 2 in, 2 out]
            n43 = call-poly <vilib>:"NT Read Value.vi"("name"="Auto_Error" ("Name")) -> ("value"=→"Auto_Error_GUI":bool)  [unwired: 8 in, 2 out]
            n44 = call-poly <vilib>:"NT Read Value.vi"("name"="Robot_is_Autonomous" ("Name")) -> ("value"=→"Robot_is_Autonomous_GUI_0" →"Robot_is_Autonomous_GUI_1" →"Robot_is_Autonomous_GUI_2":bool)  [unwired: 8 in, 2 out]
            n45 = local read "Dashboard Tab"() -> (w47:T1)
            n46 = local read "Dashboard Tab"() -> (w48:T1)
            n47 = case shown="\"Setup/Auto\"" w47 {
              frame "Checklist", Default {
              }
              frame "Setup/Auto" {
                n48 = call-poly <vilib>:"NT Read Value.vi"("default value"="No robot code versioning information..." ("Default Value"), "name"="Robot_Code_Version" ("Name")) -> ("value"=→"Robot_Code_Version_GUI":string)  [unwired: 7 in, 2 out]
              }
            }
            n49 = To Double Precision Float(number=w48) -> (double precision float=w49:dbl)
            n50 = call "ReducedBWSendToNT.vim"("Value In"=w49, "NT Name"="Dashboard_Tab" ("Name")) -> ()  [unwired: 1 out]
          }
          frame #1 {
            w90 = dbl[] [] ("default value")
            # "targeting data"
            # "report robot pose and targeting data"
            n51 = call-poly <vilib>:"NT Read Value.vi"("default value"=0.0, "name"="Alliance_Color" ("Name")) -> ("value"=w134:dbl)  [unwired: 7 in, 2 out]
            n52 = To Unsigned Word Integer(number=w134) -> (unsigned 16bit integer=w132:u16)
            n53 = call-poly <vilib>:"NT Read Value.vi"("name"="Alliance_Color" ("Name")) -> ("value"=w152:dbl)  [unwired: 8 in, 2 out]
            n54 = To Unsigned Word Integer(number=w152) -> (unsigned 16bit integer=w162:u16)
            n55 = Equal?(x=w132, y=WPI_DriverStationAllianceInfo."Red" ("x")) -> (x = y?=w125:bool)
            n56 = feedback #1(w162) -> (w158:u16)
            n57 = feedback-in #1(w162) -> ()
            n58 = Not Equal?(x=w162, y=w158) -> (x != y?=w160:bool)
            n59 = feedback #2("Field Map") -> (w163:u16)
            n60 = feedback-in #2("Field Map") -> ()
            n61 = Not Equal?(x="Field Map", y=w163) -> (x != y?=w165:bool)
            n62 = call-poly <vilib>:"NT Read Value.vi"("default value"=300.0 ("Default Value"), "name"="Field_Width" ("Name")) -> ("value"=w126:dbl)  [unwired: 7 in, 2 out]
            n63 = call-poly <vilib>:"NT Read Value.vi"("default value"=600.0 ("Default Value"), "name"="Field_Length" ("Name")) -> ("value"=w127:dbl)  [unwired: 7 in, 2 out]
            n64 = Select(t=u32 16711680 ("Color"), s=w125, f=u32 255 ("Color")) -> (s? t:f=w128:u32)
            n65 = First Call?() -> (First Call?: T/F=w159:bool)
            n66 = call "EdgeTrigger.vi"("Input Signal"="Export_Robot_Pose") -> ("Rising Edge Trigger"=w166:bool)  [unwired: 2 out]
            n67 = stacked-sequence {
              tunnel: w128 -> [w180 w182 w185]
              frame #0 {
                w181 = u32 0 ("Active Plot")
                n68 = property on="Robot Pose 2" class="XYGraph (strict)"("Active Plot"=w181, "Plot.Plot Color"=w180) -> ()  [unwired: 2 in, 2 out]
                n69 = property on="Robot Pose 1" class="XYGraph (strict)"("Active Plot"=w181, "Plot.Plot Color"=w180) -> ()  [unwired: 2 in, 2 out]
              }
              frame #1 {
                w183 = u32 1 ("Active Plot")
                n70 = property on="Robot Pose 2" class="XYGraph (strict)"("Active Plot"=w183, "Plot.Plot Color"=w182) -> ()  [unwired: 2 in, 2 out]
                n71 = property on="Robot Pose 1" class="XYGraph (strict)"("Active Plot"=w183, "Plot.Plot Color"=w182) -> ()  [unwired: 2 in, 2 out]
              }
              frame #2 {
                w184 = u32 5 ("Active Plot")
                n72 = property on="Robot Pose 2" class="XYGraph (strict)"("Active Plot"=w184, "Plot.Fill/Pt. Color"=w185) -> ()  [unwired: 2 in, 2 out]
                n73 = property on="Robot Pose 1" class="XYGraph (strict)"("Active Plot"=w184, "Plot.Fill/Pt. Color"=w185) -> ()  [unwired: 2 in, 2 out]
              }
            }
            n74 = Compound Arithmetic op=OR(w160, w159, w165) -> (w161:bool)
            n75 = property on="Robot Pose 1" class="XYGraph (strict)"("XScale.Maximum"=w126, "YScale.Maximum"=w127) -> ()  [unwired: 2 in, 2 out]
            n76 = case shown="True" w161 {
              tunnel: w162 -> [_ w192]
              tunnel: "Field Map" -> [_ w190]
              frame False {
              }
              frame True {
                # "load and display a field map"
                n77 = To Long Integer(number=w190) -> (32bit integer=w188:i32)
                n78 = Current VI's Path() -> (path=w195:path)
                n79 = Strip Path(path=w195) -> (stripped path=w194:path)  [unwired: 1 out]
                n80 = Strip Path(path=w194) -> (stripped path=w191:path)  [unwired: 1 out]
                n81 = List Folder(path=w191, pattern="*map*.png") -> (filenames=w189:string[])  [unwired: 2 in, 3 out]
                n82 = Index Array(array=w189, index=w188) -> (element=w187:string)
                n83 = property on="Field Map" class="Ring (strict)"("Strings []"=w189) -> ()  [unwired: 2 in, 2 out]
                n84 = Build Path(base path=w191, name or relative path=w187) -> (appended path=w193:path)
                n85 = call <vilib>:"Read PNG File.vi"("path to PNG file"=w193) -> ("error out"=w197:errorcluster, "image data"=w196:T20)  [unwired: 8 in, 1 out]
                n86 = case shown="No Error" w197 {
                  tunnel: w196 -> [w200 _]
                  tunnel: w192 -> [w215 _]
                  frame No Error {
                    w210 = T13 4 items=["Grayscale (U8)", "Grayscale (I16)", "Grayscale (SGL)", "Complex (CSG)", "RGB (U32)", "HSL (U32)", "RGB (U64)", "Grayscale (U16)"] ("Image Type")
                    w230 = T13 4 items=["Grayscale (U8)", "Grayscale (I16)", "Grayscale (SGL)", "Complex (CSG)", "RGB (U32)", "HSL (U32)", "RGB (U64)", "Grayscale (U16)"] ("Image Type")
                    n87 = call <vilib>:"Unflatten Pixmap.vi"("image data"=w200) -> ("24-bit pixmap"=w229:u32[][])  [unwired: 4 in, 6 out]
                    n88 = call <vilib>:"Unflatten Pixmap.vi"("image data"=w200) -> ("24-bit pixmap"=w209:u32[][])  [unwired: 4 in, 6 out]
                    n89 = property on="Robot Pose 1" class="XYGraph (strict)"() -> ("Width"=w233:u32, "Height"=w232:u32)  [unwired: 2 in, 2 out]
                    n90 = property on="Robot Pose 2" class="XYGraph (strict)"() -> ("Width"=w213:u32, "Height"=w212:u32)  [unwired: 2 in, 2 out]
                    n91 = call "IMAQ Create"("Image Name"="field1", "Image Type"=w230) -> ("New Image"=w228:T3)  [unwired: 3 in, 1 out]
                    n92 = call "IMAQ Create"("Image Name"="field2", "Image Type"=w210) -> ("New Image"=w208:T3)  [unwired: 3 in, 1 out]
                    n93 = Equal?(x=w215, y=WPI_DriverStationAllianceInfo."Red" ("x")) -> (x = y?=w217:bool)
                    n94 = call "IMAQ ArrayToColorImage"("Image Pixels (U32)"=w229, "Image"=w228) -> ("Image Out"=w227:T3)  [unwired: 3 in, 1 out]
                    n95 = call "IMAQ ArrayToColorImage"("Image Pixels (U32)"=w209, "Image"=w208) -> ("Image Out"=w207:T3)  [unwired: 3 in, 1 out]
                    n96 = To Long Integer(number=w233) -> (32bit integer=w223:i32)
                    n97 = To Long Integer(number=w232) -> (32bit integer=w224:i32)
                    n98 = To Long Integer(number=w213) -> (32bit integer=w203:i32)
                    n99 = To Long Integer(number=w212) -> (32bit integer=w204:i32)
                    n100 = call "IMAQ Resample"("X Resolution"=w223, "Y Resolution"=w224, "Image Src"=w227) -> ("Image Dst Out"=w222:T3)  [unwired: 7 in, 1 out]
                    n101 = call "IMAQ Resample"("X Resolution"=w203, "Y Resolution"=w204, "Image Src"=w207) -> ("Image Dst Out"=w202:T3)  [unwired: 7 in, 1 out]
                    n102 = Select(t=180.0, s=w217, f=0.0) -> (s? t:f=w220:dbl)
                    n103 = To Single Precision Float(number=w220) -> (single precision float=w198:sgl)
                    n104 = call "IMAQ Rotate"("Angle (degrees)"=w198, "Image Src"=w222) -> ("Image Dst Out"=w221:T3)  [unwired: 8 in, 1 out]
                    n105 = call "IMAQ Rotate"("Angle (degrees)"=w198, "Image Src"=w202) -> ("Image Dst Out"=w201:T3)  [unwired: 8 in, 1 out]
                    n106 = call "IMAQ ColorImageToArray"("Image"=w221) -> ("Image Pixels (U32)"=w226:u32[][])  [unwired: 3 in, 2 out]
                    n107 = call "IMAQ ColorImageToArray"("Image"=w201) -> ("Image Pixels (U32)"=w206:u32[][])  [unwired: 3 in, 2 out]
                    n108 = call <vilib>:"Flatten Pixmap.vi"("24-bit pixmap"=w226) -> ("image data"=w225:T20)  [unwired: 10 in]
                    n109 = call <vilib>:"Flatten Pixmap.vi"("24-bit pixmap"=w206) -> ("image data"=w205:T20)  [unwired: 10 in]
                    n110 = call <vilib>:"Draw Flattened Pixmap.vi"("image data"=w225) -> ("new picture"=w214:picture)  [unwired: 8 in]
                    n111 = call <vilib>:"Draw Flattened Pixmap.vi"("image data"=w205) -> ("new picture"=w199:picture)  [unwired: 8 in]
                    n112 = property on="Robot Pose 1" class="XYGraph (strict)"("PlotImages.Back"=w214) -> ()  [unwired: 2 in, 2 out]
                    n113 = property on="Robot Pose 2" class="XYGraph (strict)"("PlotImages.Back"=w199) -> ()  [unwired: 2 in, 2 out]
                  }
                  frame Error {
                  }
                }
              }
            }
            n114 = case shown="True" w166 {
              frame False {
              }
              frame True {
                # "export the current robot pose data"
                n115 = Get Date/Time In Seconds() -> (seconds since 1Jan1904=w247:timestamp)
                n116 = Format Date/Time String(time format string (%c)="%Y-%m-%d_%H-%M", seconds (now)=w247) -> (date/time string=w245:string)  [unwired: 1 in]
                n117 = Concatenate Strings("robot pose data " ("string"), w245) -> (w243:string)
                n118 = Current VI's Path() -> (path=w242:path)
                n119 = String To Path(string=w243) -> (path=w239:path)
                n120 = Strip Path(path=w242) -> (stripped path=w241:path)  [unwired: 1 out]
                n121 = Strip Path(path=w241) -> (stripped path=w240:path)  [unwired: 1 out]
                n122 = Build Path(base path=w240, name or relative path=w239) -> (appended path=w238:path)
                n123 = invoke on="Robot Pose 1" class="XYGraph (strict)" method="Export Image"("FileType"=enum32{"BMP", "EPS", "EMF", "PICT"}."BMP" ("File Type"), "Target"=enum32{"File", "Clipboard"}."File", "Path"=w238, "HideGrid"=TRUE ("Hide Grid"), "Overwrite"=TRUE ("Always Overwrite")) -> ()  [unwired: 3 in, 8 out]
              }
            }
            n124 = property on="Robot Pose 2" class="XYGraph (strict)"("XScale.Maximum"=w126, "YScale.Maximum"=w127) -> ()  [unwired: 2 in, 2 out]
            n125 = call-poly <vilib>:"NT Read Value.vi"("default value"=0.0 ("Default Value"), "name"="Robot_P" ("Name")) -> ("value"=→"Robot_P":dbl)  [unwired: 7 in, 2 out]
            n126 = call-poly <vilib>:"NT Read Value.vi"("default value"=0.0 ("Default Value"), "name"="Robot_H" ("Name")) -> ("value"=w177:dbl)  [unwired: 7 in, 2 out]
            n127 = call-poly <vilib>:"NT Read Value.vi"("default value"=-1.0 ("Default Value"), "name"="Robot_Y" ("Name")) -> ("value"=w123:dbl)  [unwired: 7 in, 2 out]
            "Robot_Y" <- w123
            n128 = call-poly <vilib>:"NT Read Value.vi"("default value"=-1.0 ("Default Value"), "name"="Robot_X" ("Name")) -> ("value"=w122:dbl)  [unwired: 7 in, 2 out]
            "Robot_X" <- w122
            n129 = call-poly <vilib>:"NT Read Value.vi"("default value"=dbl[] [0.0, 0.0, 0.0, 0.0] ("Default Value"), "name"="Targeting_Information" ("Name")) -> ("value"=w124:dbl[])  [unwired: 7 in, 2 out]
            n130 = call-poly <vilib>:"NT Read Value.vi"("default value"=30.0 ("Default Value"), "name"="Robot_Width_Bumpers" ("Name")) -> ("value"=w146:dbl)  [unwired: 7 in, 2 out]
            n131 = call-poly <vilib>:"NT Read Value.vi"("default value"=30.0 ("Default Value"), "name"="Robot_Length_Bumpers" ("Name")) -> ("value"=w147:dbl)  [unwired: 7 in, 2 out]
            n132 = Quotient & Remainder(x=w177, y=360.0) -> (x-y*floor(x/y)=→"Robot_H_GUI":dbl)  [unwired: 1 out]
            n133 = call-poly <vilib>:"NT Read Value.vi"("default value"=w90, "name"="Auto_Path_Xs" ("Name")) -> ("value"=w91:dbl[])  [unwired: 7 in, 2 out]
            n134 = call-poly <vilib>:"NT Read Value.vi"("default value"=w90, "name"="Auto_Path_Ys" ("Name")) -> ("value"=w93:dbl[])  [unwired: 7 in, 2 out]
            n135 = Bundle("value"=w93, "value"=w91) -> (w95:cluster{"value":dbl[], "value":dbl[]})  [unwired: 1 in]
            n136 = call "RenderRobotPose.vi"("Robot X (in)"=w122, "Robot Width (in)"=w146, "Robot Length (in)"=w147, "Buffer Time (min)"=0.5, "Robot Y (in)"=w123, "Targeting Information"=w124, "Robot Heading (deg)"=w177, "Planned Path"=w95, "Robot Enabled"=TRUE, "Reset"="Clear_Robot_Pose_Display") -> ("Robot Pose"=→"Robot Pose 2" →"Robot Pose 1":cluster{dbl[], dbl[]}[])  [unwired: 5 in]
            n137 = local read "No_Secondary_Camera"() -> (w140:bool)
            n138 = property on="Robot Pose 2" class="XYGraph (strict)"("Visible"=w140) -> ()  [unwired: 2 in, 2 out]
            n139 = call-poly <vilib>:"NT Read Value.vi"("default value"=FALSE, "name"="Pointed_at_Target" ("Name")) -> ("value"=→"Pointed_at_Target":bool)  [unwired: 7 in, 2 out]
            n140 = call-poly <vilib>:"NT Read Value.vi"("name"="LL_Valid" ("Name")) -> ("value"=→"LL_Valid":bool)  [unwired: 8 in, 2 out]
            n141 = call-poly <vilib>:"NT Read Value.vi"("name"="Vision_Fault" ("Name")) -> ("value"=→"Vision_Fault_GUI":bool)  [unwired: 8 in, 2 out]
            n142 = call-poly <vilib>:"NT Read Value.vi"("default value"=0.0, "name"="Distance_to_Target" ("Name")) -> ("value"=→"Distance_to_Target":dbl)  [unwired: 7 in, 2 out]
            n143 = call-poly <vilib>:"NT Read Value.vi"("default value"=0.0, "name"="Heading_to_Target" ("Name")) -> ("value"=→"Heading_to_Target":dbl)  [unwired: 7 in, 2 out]
            n144 = call-poly <vilib>:"NT Read Value.vi"("default value"=0.0, "name"="TOF_Range" ("Name")) -> ("value"=→"TOF_Range":dbl)  [unwired: 7 in, 2 out]
            n145 = call "ReducedBWSendToNT.vim"("Value In"="New_Blue_Calibration", "NT Name"="New_Blue_Calibration") -> ()  [unwired: 1 out]
            n146 = call-poly <vilib>:"NT Read Value.vi"("default value"=0.0, "name"="Current_Blue_Calibration" ("NT Name")) -> ("value"=w96:dbl)  [unwired: 7 in, 2 out]
            "Current_Blue_Calibration" <- w96
            n147 = call "ReducedBWSendToNT.vim"("Value In"="New_Red_Calibration", "NT Name"="New_Red_Calibration") -> ()  [unwired: 1 out]
            n148 = call "ReducedBWSendToNT.vim"("Value In"="Apply_Grid_Calibration", "NT Name"="Apply_Grid_Calibration") -> ()  [unwired: 1 out]
            n149 = call-poly <vilib>:"NT Read Value.vi"("default value"=0.0, "name"="Current_Red_Calibration" ("NT Name")) -> ("value"=w102:dbl)  [unwired: 7 in, 2 out]
            "Current_Red_Calibration" <- w102
            n150 = call "Is Value Changed.vim"("value"=w96) -> ("changed or first call?"=w97:bool)
            n151 = call "Is Value Changed.vim"("value"=w102) -> ("changed or first call?"=w103:bool)
            n152 = case shown="True" w97 {
              tunnel: w96 -> [_ w178]
              frame False {
              }
              frame True {
                n153 = property on="New_Blue_Calibration" class="DigNum (strict)"("Value"=w178) -> ()  [unwired: 2 in, 2 out]
              }
            }
            n154 = case shown="True" w103 {
              tunnel: w102 -> [_ w179]
              frame False {
              }
              frame True {
                n155 = property on="New_Red_Calibration" class="DigNum (strict)"("Value"=w179) -> ()  [unwired: 2 in, 2 out]
              }
            }
          }
          frame #2 {
            # "driver control configuration"
            # "robot configuration"
            # "robot and driver control configuration"
            n156 = local read "Dashboard Tab"() -> (w248:T1)
            n157 = case shown="\"Setup/Auto\"" w248 {
              frame "Checklist", Default {
              }
              frame "Setup/Auto" {
                n158 = call-poly <vilib>:"NT Read Value.vi"("default value"="No robot profile..." ("Default Value"), "name"="Robot_Profile" ("Name")) -> ("value"=→"Robot_Profile_GUI":string)  [unwired: 7 in, 2 out]
              }
            }
            n159 = Build Array("N/A") -> (w259:string[])
            n160 = And(x="Calibrate_Joysticks_GUI", y="Arm_Calibrate_Joysticks") -> (x .and. y?=w249:bool)
            n161 = To Double Precision Float(number="Select Driver Profile") -> (double precision float=w252:dbl)
            n162 = call-poly <vilib>:"NT Read Value.vi"("default value"=w259, "name"="Legal_Drivers" ("Name")) -> ("value"=w258:string[])  [unwired: 7 in, 2 out]
            "Legal_Drivers_GUI" <- w258
            n163 = Not(x="Arm_Calibrate_Joysticks") -> (.not. x?=w261:bool)
            n164 = call "ReducedBWSendToNT.vim"("Value In"=w252, "NT Name"="Selected_Driver" ("Name")) -> ()  [unwired: 1 out]
            n165 = property on="Select Driver Profile" class="Ring (strict)"("Strings []"=w258) -> ()  [unwired: 2 in, 2 out]
            n166 = call "ReducedBWSendToNT.vim"("Value In"=w249, "NT Name"="Calibrate_Joysticks" ("Name")) -> ()  [unwired: 1 out]
            n167 = Select(t=cluster{u32, u32}[] [{11776947, 16448250}, {16448250, 16448250}] ("Colors [4]"), s=w261, f=cluster{u32, u32}[] [{6618880, 16448250}, {16448250, 16448250}] ("Colors [4]")) -> (s? t:f=w262:cluster{u32, u32}[])
            n168 = property on="Calibrate_Joysticks_GUI" class="Bool"("Colors [4]"=w262) -> ()  [unwired: 2 in, 2 out]
          }
          frame #3 {
            # "configure auto play"
            # "set robot pose"
            # "autonomous configuration"
            n169 = call "ReducedBWSendToNT.vim"("Value In"="Manual_Start_X", "NT Name"="Manual_Start_X" ("Name")) -> ()  [unwired: 1 out]
            n170 = call "ReducedBWSendToNT.vim"("Value In"="Manual_Start_Y", "NT Name"="Manual_Start_Y" ("Name")) -> ()  [unwired: 1 out]
            n171 = call "ReducedBWSendToNT.vim"("Value In"="Manual_Start_H", "NT Name"="Manual_Start_H" ("Name")) -> ()  [unwired: 1 out]
            n172 = call "ReducedBWSendToNT.vim"("Value In"="Disable_Fusion_While_Autonomous", "NT Name"="Disable_Fusion_While_Autonomous" ("Name")) -> ()  [unwired: 1 out]
            n173 = call "ReducedBWSendToNT.vim"("Value In"="Disable_Fusion_While_Disabled", "NT Name"="Disable_Fusion_While_Disabled" ("Name")) -> ()  [unwired: 1 out]
            n174 = call "ReducedBWSendToNT.vim"("Value In"="Push_Robot_Start_GUI", "NT Name"="Push_Robot_Start" ("Name")) -> ()  [unwired: 1 out]
            n175 = local read "Dashboard Tab"() -> (w269:T1)
            n176 = To Double Precision Float(number="Select Autonomous Play") -> (double precision float=w272:dbl)
            n177 = call "ReducedBWSendToNT.vim"("Value In"="Auto_Test_Mode_GUI", "NT Name"="Auto_Test_Mode" ("Name")) -> ()  [unwired: 1 out]
            n178 = call "ReducedBWSendToNT.vim"("Value In"="Auto_Delay_GUI", "NT Name"="Auto_Delay" ("Name")) -> ()  [unwired: 1 out]
            n179 = call "ReducedBWSendToNT.vim"("Value In"="Force_Human_Control_GUI", "NT Name"="Force_Human_Control" ("Name")) -> ()  [unwired: 1 out]
            n180 = call "ReducedBWSendToNT.vim"("Value In"=w272, "NT Name"="Selected_Auto_Play" ("Name")) -> ()  [unwired: 1 out]
            n181 = call "ReducedBWSendToNT.vim"("Value In"="Refresh_Auto_Play_List_GUI", "NT Name"="Refresh_Auto_Play_List" ("Name")) -> ()  [unwired: 1 out]
            n182 = case shown="\"Setup/Auto\"" w269 {
              tunnel: "Select Autonomous Play" -> [_ w292]
              tunnel: "Refresh_Auto_Play_List_GUI" -> [_ w291]
              frame "Checklist", Default {
              }
              frame "Setup/Auto" {
                w309 = "N/A" ("Default Value")
                n183 = call-poly <vilib>:"NT Read Value.vi"("default value"=0.0, "name"="Suggested_Start_H" ("Name")) -> ("value"=w308:dbl)  [unwired: 7 in, 2 out]
                n184 = call-poly <vilib>:"NT Read Value.vi"("default value"=0.0, "name"="Suggested_Start_X" ("Name")) -> ("value"=w306:dbl)  [unwired: 7 in, 2 out]
                n185 = call-poly <vilib>:"NT Read Value.vi"("default value"=0.0, "name"="Suggested_Start_Y" ("Name")) -> ("value"=w307:dbl)  [unwired: 7 in, 2 out]
                n186 = Build Array("N/A") -> (w312:string[])
                n187 = call "Is Value Changed.vim"("value"=w292) -> ("changed or first call?"=w293:bool)
                n188 = call "Is Value Changed.vim"("value"=w308) -> ("changed or first call?"=w299:bool)
                n189 = call "Is Value Changed.vim"("value"=w306) -> ("changed or first call?"=w295:bool)
                n190 = call "Is Value Changed.vim"("value"=w307) -> ("changed or first call?"=w297:bool)
                n191 = call-poly <vilib>:"NT Read Value.vi"("default value"=w309, "name"="Auto_Playbook" ("Name")) -> ("value"=→"Auto_Playbook_GUI":string)  [unwired: 7 in, 2 out]
                n192 = call-poly <vilib>:"NT Read Value.vi"("default value"=w309, "name"="Auto_Path_Suffix" ("Name")) -> ("value"=→"Auto_Suffix_GUI":string)  [unwired: 7 in, 2 out]
                n193 = call-poly <vilib>:"NT Read Value.vi"("default value"=w312, "name"="Legal_Auto_Plays" ("Name")) -> ("value"=w313:string[])  [unwired: 7 in, 2 out]
                n194 = Compound Arithmetic op=OR(w293, w291, w295) -> (w294:bool)
                n195 = Compound Arithmetic op=OR(w293, w291, w297) -> (w296:bool)
                n196 = Compound Arithmetic op=OR(w293, w291, w299) -> (w298:bool)
                n197 = property on="Select Autonomous Play" class="Ring (strict)"("Strings []"=w313) -> ()  [unwired: 2 in, 2 out]
                n198 = case shown="True" w298 {
                  tunnel: w308 -> [_ w318]
                  frame False {
                  }
                  frame True {
                    n199 = property on="Manual_Start_H" class="DigNum (strict)"("Value"=w318) -> ()  [unwired: 2 in, 2 out]
                  }
                }
                n200 = case shown="True" w296 {
                  tunnel: w307 -> [_ w319]
                  frame False {
                  }
                  frame True {
                    n201 = property on="Manual_Start_Y" class="DigNum (strict)"("Value"=w319) -> ()  [unwired: 2 in, 2 out]
                  }
                }
                n202 = case shown="True" w294 {
                  tunnel: w306 -> [_ w320]
                  frame False {
                  }
                  frame True {
                    n203 = property on="Manual_Start_X" class="DigNum (strict)"("Value"=w320) -> ()  [unwired: 2 in, 2 out]
                  }
                }
              }
            }
          }
          frame #4 {
            # "scoring states"
            # "master state controller"
            # "state indicators"
          }
          frame #5 {
            # "actuator test interlocks"
            # "emergency overrides"
            # "emergency overrides and interlocks"
            n204 = global read "GlobalDashboard.vi" "Code_is_Running"() -> (w324:bool)
            n205 = call-poly <vilib>:"NT Read Value.vi"("default value"=FALSE, "name"="Robot_in_Safety_Override" ("Name")) -> ("value"=w326:bool)  [unwired: 7 in, 2 out]
            n206 = call "EdgeTrigger.vi"("Input Signal"=w326) -> ("All Edge Trigger"=w327:bool)  [unwired: 2 out]
            n207 = call "EdgeTrigger.vi"("Input Signal"=w324) -> ("Falling Edge Trigger"=w323:bool)  [unwired: 2 out]
            n208 = call "ReducedBWSendToNT.vim"("Value In"="Clear_Errors_GUI", "NT Name"="Clear_Errors" ("Name")) -> ()  [unwired: 1 out]
            n209 = call "ReducedBWSendToNT.vim"("Value In"="Super_Test_Mode_GUI", "NT Name"="Super_Test_Mode" ("Name")) -> ()  [unwired: 1 out]
            n210 = call "ReducedBWSendToNT.vim"("Value In"="Auto_Targeting_Override", "NT Name"="Auto_Targeting_Override" ("Name")) -> ()  [unwired: 1 out]
            n211 = call "ReducedBWSendToNT.vim"("Value In"="Camera_Override_GUI", "NT Name"="Camera_Override" ("Name")) -> ()  [unwired: 1 out]
            n212 = call "ReducedBWSendToNT.vim"("Value In"="Field_Oriented_Override_GUI", "NT Name"="Field_Oriented_Override" ("Name")) -> ()  [unwired: 1 out]
            n213 = case shown="True" w327 {
              tunnel: w326 -> [_ w352]
              frame False {
              }
              frame True {
                n214 = property on="Master_Safety_Override_1" class="Bool (strict)"("Value"=w352) -> ()  [unwired: 2 in, 2 out]
              }
            }
            n215 = case shown="True" w323 {
              frame False {
              }
              frame True {
                n216 = property on="Master_Safety_Override_1" class="Bool (strict)"("Value"=FALSE ("Master_Safety_Override_1")) -> ()  [unwired: 2 in, 2 out]
              }
            }
            n217 = call "ReducedBWSendToNT.vim"("Value In"="Master_Safety_Override_1", "NT Name"="Master_Safety_Override" ("Name")) -> ()  [unwired: 1 out]
            n218 = property on="Actuator Testing" class="Ring (strict)"() -> ("RingText.Text"=w336:string)  [unwired: 2 in, 2 out]
            n219 = Build Array("No_Test") -> (w350:string[])
            n220 = call "ReducedBWSendToNT.vim"("Value In"="Free_Tuning_Variable_GUI", "NT Name"="Free_Tuning_Variable" ("Name")) -> ()  [unwired: 1 out]
            n221 = call-poly <vilib>:"NT Read Value.vi"("default value"=w350, "name"="Legal_Actuator_Names" ("Name")) -> ("value"=w349:string[])  [unwired: 7 in, 2 out]
            n222 = call "ReducedBWSendToNT.vim"("Value In"=w336, "NT Name"="Test_Actuator_Name" ("Name")) -> ()  [unwired: 1 out]
            n223 = call "ReducedBWSendToNT.vim"("Value In"="Test_Actuator_Value_GUI", "NT Name"="Test_Actuator_Value" ("Name")) -> ()  [unwired: 1 out]
            n224 = call "ReducedBWSendToNT.vim"("Value In"="Test_Actuator_Period_GUI", "NT Name"="Test_Actuator_Period" ("Name")) -> ()  [unwired: 1 out]
            n225 = property on="Actuator Testing" class="Ring (strict)"("Strings []"=w349) -> ()  [unwired: 2 in, 2 out]
          }
          frame #6 {
            # "drivebase subsytem"
            n226 = call "SwerveModuleReadData.vi"("NT Name (Errors)"="Swerve_1_Errors", "NT Name (Details)"="Swerve_1_Details" ("NT Name (Tune)")) -> ("Shifter State"=→"Swerve_1_Shifter_State":string, "Drive Velocity"=→"Swerve_1_Drive_Velocity":dbl, "Drive Temperature"=→"Swerve_1_Drive_Temperature":dbl, "Azimuth Position"=→"Swerve_1_Azimuth_Position":dbl, "Shifter Failure"=w419:T21, "Drive Overheating"=w421:T21, "Drive Fault"=w366:T21, "Azimuth Fault"=w420:T21)  [unwired: 2 in]
            n227 = call "SwerveModuleReadData.vi"("NT Name (Errors)"="Swerve_0_Errors", "NT Name (Details)"="Swerve_0_Details" ("NT Name (Tune)")) -> ("Shifter State"=→"Swerve_0_Shifter_State":string, "Drive Velocity"=→"Swerve_0_Drive_Velocity":dbl, "Drive Temperature"=→"Swerve_0_Drive_Temperature":dbl, "Azimuth Position"=→"Swerve_0_Azimuth_Position":dbl, "Shifter Failure"=w427:T21, "Drive Overheating"=w435:T21, "Drive Fault"=w368:T21, "Azimuth Fault"=w431:T21)  [unwired: 2 in]
            n228 = call-poly <vilib>:"NT Read Value.vi"("name"="IMU_Failure" ("Name")) -> ("value"=→"IMU_Failure_GUI":bool)  [unwired: 8 in, 2 out]
            n229 = call-poly <vilib>:"NT Read Value.vi"("name"="Field_Oriented" ("Name")) -> ("value"=→"Field_Oriented_GUI":bool)  [unwired: 8 in, 2 out]
            n230 = call "SwerveModuleReadData.vi"("NT Name (Errors)"="Swerve_2_Errors", "NT Name (Details)"="Swerve_2_Details" ("NT Name (Tune)")) -> ("Shifter State"=→"Swerve_2_Shifter_State":string, "Drive Velocity"=→"Swerve_2_Drive_Velocity":dbl, "Drive Temperature"=→"Swerve_2_Drive_Temperature":dbl, "Azimuth Position"=→"Swerve_2_Azimuth_Position":dbl, "Shifter Failure"=w414:T21, "Drive Overheating"=w416:T21, "Drive Fault"=w364:T21, "Azimuth Fault"=w415:T21)  [unwired: 2 in]
            n231 = call "SwerveModuleReadData.vi"("NT Name (Errors)"="Swerve_3_Errors", "NT Name (Details)"="Swerve_3_Details" ("NT Name (Tune)")) -> ("Shifter State"=→"Swerve_3_Shifter_State":string, "Drive Velocity"=→"Swerve_3_Drive_Velocity":dbl, "Drive Temperature"=→"Swerve_3_Drive_Temperature":dbl, "Azimuth Position"=→"Swerve_3_Azimuth_Position":dbl, "Shifter Failure"=w409:T21, "Drive Overheating"=w411:T21, "Drive Fault"=w362:T21, "Azimuth Fault"=w410:T21)  [unwired: 2 in]
            n232 = Unbundle(w421) -> ("Boolean"=w407:bool, "Numeric Text.Text Colors:Text Color"=w404:u32)
            n233 = Unbundle(w420) -> ("Boolean"=w408:bool, "Numeric Text.Text Colors:Text Color"=w405:u32)
            n234 = Unbundle(w435) -> ("Boolean"=w433:bool, "Numeric Text.Text Colors:Text Color"=w434:u32)
            n235 = Unbundle(w431) -> ("Boolean"=w430:bool, "Numeric Text.Text Colors:Text Color"=w428:u32)
            n236 = Unbundle(w419) -> ("Boolean"=w406:bool, "Numeric Text.Text Colors:Text Color"=w399:u32)
            n237 = Unbundle(w416) -> ("Boolean"=w397:bool, "Numeric Text.Text Colors:Text Color"=w395:u32)
            n238 = Unbundle(w427) -> ("Boolean"=w425:bool, "Numeric Text.Text Colors:Text Color"=w426:u32)
            n239 = Unbundle(w368) -> ("Boolean"=w360:bool, "Numeric Text.Text Colors:Text Color"=w369:u32)
            n240 = Unbundle(w415) -> ("Boolean"=w398:bool, "Numeric Text.Text Colors:Text Color"=w396:u32)
            n241 = Unbundle(w411) -> ("Boolean"=w386:bool, "Numeric Text.Text Colors:Text Color"=w385:u32)
            n242 = Unbundle(w410) -> ("Boolean"=w387:bool, "Numeric Text.Text Colors:Text Color"=w388:u32)
            n243 = Unbundle(w366) -> ("Boolean"=w359:bool, "Numeric Text.Text Colors:Text Color"=w367:u32)
            n244 = Unbundle(w414) -> ("Boolean"=w390:bool, "Numeric Text.Text Colors:Text Color"=w389:u32)
            n245 = Unbundle(w364) -> ("Boolean"=w358:bool, "Numeric Text.Text Colors:Text Color"=w365:u32)
            n246 = Unbundle(w409) -> ("Boolean"=w379:bool, "Numeric Text.Text Colors:Text Color"=w380:u32)
            n247 = Unbundle(w362) -> ("Boolean"=w357:bool, "Numeric Text.Text Colors:Text Color"=w363:u32)
            n248 = property on="Swerve_3_Drive_Velocity" class="DigNum (strict)"("NumText.BG Color"=w363) -> ()  [unwired: 2 in, 2 out]
            n249 = property on="Swerve_0_Azimuth_Position" class="DigNum (strict)"("NumText.BG Color"=w428) -> ()  [unwired: 2 in, 2 out]
            n250 = property on="Swerve_0_Drive_Temperature" class="DigNum (strict)"("NumText.BG Color"=w434) -> ()  [unwired: 2 in, 2 out]
            n251 = property on="Swerve_0_Shifter_State" class="Str"("Text.BG Color"=w426) -> ()  [unwired: 2 in, 2 out]
            n252 = property on="Swerve_1_Azimuth_Position" class="DigNum (strict)"("NumText.BG Color"=w405) -> ()  [unwired: 2 in, 2 out]
            n253 = property on="Swerve_1_Drive_Temperature" class="DigNum (strict)"("NumText.BG Color"=w404) -> ()  [unwired: 2 in, 2 out]
            n254 = property on="Swerve_1_Shifter_State" class="Str"("Text.BG Color"=w399) -> ()  [unwired: 2 in, 2 out]
            n255 = property on="Swerve_2_Azimuth_Position" class="DigNum (strict)"("NumText.BG Color"=w396) -> ()  [unwired: 2 in, 2 out]
            n256 = property on="Swerve_2_Drive_Temperature" class="DigNum (strict)"("NumText.BG Color"=w395) -> ()  [unwired: 2 in, 2 out]
            n257 = property on="Swerve_2_Shifter_State" class="Str"("Text.BG Color"=w389) -> ()  [unwired: 2 in, 2 out]
            n258 = property on="Swerve_3_Azimuth_Position" class="DigNum (strict)"("NumText.BG Color"=w388) -> ()  [unwired: 2 in, 2 out]
            n259 = property on="Swerve_3_Drive_Temperature" class="DigNum (strict)"("NumText.BG Color"=w385) -> ()  [unwired: 2 in, 2 out]
            n260 = property on="Swerve_3_Shifter_State" class="Str"("Text.BG Color"=w380) -> ()  [unwired: 2 in, 2 out]
            n261 = property on="Swerve_0_Drive_Velocity" class="DigNum (strict)"("NumText.BG Color"=w369) -> ()  [unwired: 2 in, 2 out]
            n262 = property on="Swerve_2_Drive_Velocity" class="DigNum (strict)"("NumText.BG Color"=w365) -> ()  [unwired: 2 in, 2 out]
            n263 = property on="Swerve_1_Drive_Velocity" class="DigNum (strict)"("NumText.BG Color"=w367) -> ()  [unwired: 2 in, 2 out]
            n264 = call-poly <vilib>:"NT Read Value.vi"("name"="Using_Auto_Targeting" ("Name")) -> ("value"=→"Using_Auto_Targeting":bool)  [unwired: 8 in, 2 out]
            n265 = Build Array(w425, w406, w390, w379) -> (→"Swerve_Shifter_Failure_Array":bool[])
            n266 = Build Array(w430, w408, w398, w387) -> (→"Swerve_Azimuth_Fault_Array":bool[])
            n267 = Build Array(w433, w407, w397, w386) -> (→"Swerve_Overheating_Array":bool[])
            n268 = Build Array(w360, w359, w358, w357) -> (→"Swerve_Drive_Fault_Array":bool[])
            n269 = local read "Dashboard Tab"() -> (w370:T1)
            n270 = case shown="\"Tune\"" w370 {
              frame "Checklist", Default {
              }
              frame "Tune" {
                n271 = call-poly <vilib>:"NT Read Value.vi"("default value"=dbl[] [0.0, 0.0, 0.0, 0.0, 0.0, 0.0] ("Default Value"), "name"="Current_Driver_Profile_Setpoints" ("Name")) -> ("value"=w460:dbl[])  [unwired: 7 in, 2 out]
                n272 = Array To Cluster(array=w460) -> (cluster=w456:T22)
                "Current_Driver_Profile_Setpoints_GUI" <- w456
                n273 = feedback #3(dbl[] [0.0, 0.0, 0.0, 0.0, 0.0, 0.0] ("Default Value")) -> (w459:dbl[])
                n274 = feedback-in #3(w460) -> ()
                n275 = Not Equal?(x=w460, y=w459) -> (x != y?=w458:bool[])
                n276 = Or Array Elements(Boolean array=w458) -> (logical OR=w457:bool)
                n277 = case shown="True" w457 {
                  tunnel: w456 -> [_ w464]
                  frame False {
                  }
                  frame True {
                    n278 = property on="New_Driver_Profile_Setpoints_GUI" class="Clust (strict)"("Value"=w464) -> ()  [unwired: 2 in, 2 out]
                  }
                }
              }
            }
            n279 = local read "Select Driver Profile"() -> (w444:u16)
            n280 = local read "Legal_Drivers_GUI"() -> (w445:string[])
            n281 = Cluster To Array(cluster="New_Driver_Profile_Setpoints_GUI") -> (array=w374:dbl[])
            n282 = And(x="Calibrate_Wheels_GUI", y="Arm_Calibrate_Wheels_GUI") -> (x .and. y?=w377:bool)
            n283 = Not(x="Arm_Calibrate_Wheels_GUI") -> (.not. x?=w451:bool)
            n284 = To Long Integer(number=w444) -> (32bit integer=w442:i32)
            n285 = call "ReducedBWSendToNT.vim"("Value In"="Home_Wheels_GUI", "NT Name"="Home_Wheels" ("Name")) -> ()  [unwired: 1 out]
            n286 = Index Array(array=w445, index=w442) -> (element=→"Current_Driver_Profile_GUI":string)
            n287 = call "ReducedBWSendToNT.vim"("Value In"="Apply_Driver_Profile_Setpoints_GUI", "NT Name"="Apply_Driver_Profile_Setpoints" ("Name")) -> ()  [unwired: 1 out]
            n288 = call "ReducedBWSendToNT.vim"("Value In"=w374, "NT Name"="New_Driver_Profile_Setpoints" ("Name")) -> ()  [unwired: 1 out]
            n289 = call "ReducedBWSendToNT.vim"("Value In"=w377, "NT Name"="Calibrate_Wheels" ("Name")) -> ()  [unwired: 1 out]
            n290 = call "ReducedBWSendToNT.vim"("Value In"="Arm_Calibrate_Wheels_GUI", "NT Name"="Unlock_Azimuth") -> ()  [unwired: 1 out]
            n291 = Select(t=cluster{u32, u32}[] [{11776947, 16448250}, {16448250, 16448250}] ("Colors [4]"), s=w451, f=cluster{u32, u32}[] [{6618880, 16448250}, {16448250, 16448250}] ("Colors [4]")) -> (s? t:f=w450:cluster{u32, u32}[])
            n292 = property on="Calibrate_Wheels_GUI" class="Bool"("Colors [4]"=w450) -> ()  [unwired: 2 in, 2 out]
          }
          frame #7 {
            # "hybrid node indicators"
            # "combine errors for in-match reporting"
            # "manage targeting reticules"
            # "manage audible warnings"
            # "error management and driver assistance"
            n293 = local read "Swerve_Azimuth_Fault_Array"() -> (w491:bool[])
            n294 = local read "Swerve_Shifter_Failure_Array"() -> (w494:bool[])
            n295 = local read "Swerve_Overheating_Array"() -> (w492:bool[])
            n296 = local read "Swerve_Drive_Fault_Array"() -> (w470:bool[])
            n297 = Or Array Elements(Boolean array=w491) -> (logical OR=→"Swerve_Azimuth_Fault":bool)
            n298 = Or Array Elements(Boolean array=w492) -> (logical OR=→"Swerve_Overheating":bool)
            n299 = Or Array Elements(Boolean array=w494) -> (logical OR=→"Swerve_Shifter_Failure":bool)
            n300 = Or Array Elements(Boolean array=w470) -> (logical OR=→"Swerve_Drive_Fault":bool)
            n301 = Build Array("Driver_Help", "Manipulator_Help") -> (w499:bool[])
            n302 = Or Array Elements(Boolean array=w499) -> (logical OR=w490:bool)
            n303 = Not(x=w490) -> (.not. x?=w507:bool)
            n304 = Build Array (concatenate)(w507, w499) -> (w506:bool[])
            n305 = property on="Help Graphic" class="ImageControl"("Visible"=w490) -> ()  [unwired: 2 in, 2 out]
            n306 = call "StateSelection.vi"("Disallowed States"=bool[] [FALSE, FALSE, FALSE, FALSE], "State Triggers"=w506, "State Names"=string[] ["No Help", "Driver Help", "Manipulator Help"]) -> ("Selected State"=w511:string)
            n307 = case shown="\"Driver Help\"" w511 {
              tunnel: [_ w532 w534] -> w493
              tunnel: w490 -> [_ _ _]
              frame "No Help", Default {
              }
              frame "Driver Help" {
                n308 = call "RenderJoystickDiagram.vi"("Joystick Graphic Filename"="driver joystick diagram.png") -> ("Image Out"=w532:T3)  [unwired: 10 in]
              }
              frame "Manipulator Help" {
                n309 = call "RenderJoystickDiagram.vi"("Joystick Graphic Filename"="manipulator joystick diagram.png") -> ("Image Out"=w534:T3)  [unwired: 10 in]
              }
            }
            "Help Graphic" <- w493
            n310 = Or Array Elements(Boolean array=w499) -> (logical OR=w501:bool)
            n311 = Not(x=w501) -> (.not. x?=w500:bool)
            n312 = Or(x=w500, y=w499) -> (x .or. y?=w498:bool[])
            n313 = Index Array(array=w498) -> (element #1=w472:bool, element #2=w471:bool)  [unwired: 2 in]
            n314 = Select(t=T15."Enabled" ("Disabled"), s=w471, f=T15."Disabled and Grayed Out" ("Disabled")) -> (s? t:f=w502:T15)
            n315 = Select(t=T15."Enabled" ("Disabled"), s=w472, f=T15."Disabled and Grayed Out" ("Disabled")) -> (s? t:f=w531:T15)
            n316 = property on="Driver_Help" class="Bool (strict)"("DisabledEnum"=w531) -> ()  [unwired: 2 in, 2 out]
            n317 = property on="Manipulator_Help" class="Bool (strict)"("DisabledEnum"=w502) -> ()  [unwired: 2 in, 2 out]
            n318 = First Call?() -> (First Call?: T/F=w479:bool)
            n319 = call-poly <vilib>:"NT Read Value.vi"("default value"=FALSE ("Default Value"), "name"="Master_Alarm" ("Name")) -> ("value"=w475:bool)  [unwired: 7 in, 2 out]
            n320 = call "Timer.vi"("Reset Timer"=w479) -> ("Time (ms)"=w478:u32)
            n321 = Greater?(x=w478, y=u32 2500) -> (0:w476:bool)
            n322 = local read "Arm_Calibrate_Wheels_GUI"() -> (w481:bool)
            n323 = call-poly <vilib>:"NT Read Value.vi"("default value"=0.0 ("Default Value"), "name"="Number_of_Master_Alarms" ("Name")) -> ("value"=w485:dbl)  [unwired: 7 in, 2 out]
            n324 = And(x=w476, y=w475) -> (x .and. y?=w474:bool)
            n325 = call "EdgeTrigger.vi"("Input Signal"="Mute_Audible_Warnings") -> ("Rising Edge Trigger"=w519:bool)  [unwired: 2 out]
            n326 = local read "Arm_Calibrate_Joysticks"() -> (w482:bool)
            n327 = To Long Integer(number=w485) -> (32bit integer=w484:i32)
            n328 = call "BlinkLight.vi"() -> ("Blinked"=w524:bool)  [unwired: 1 in]
            n329 = Number To Decimal String(number=w484) -> (decimal integer string=w525:string)  [unwired: 1 in]
            n330 = feedback #4(TRUE ("t")) -> (w517:bool)
            n331 = Not(x=w517) -> (.not. x?=w516:bool)
            n332 = Select(t=w516, s=w519, f=w517) -> (s? t:f=w473:bool)
            "Audible_Warnings_Enabled_GUI" <- w473
            n333 = feedback-in #4(w473) -> ()
            n334 = Select(t=w524, s=w474, f=FALSE) -> (s? t:f=w528:bool)
            "Master_Caution_GUI_1" <- w528
            "Master_Caution_GUI_0" <- w528
            "Master_Caution_GUI_2" <- w528
            n335 = Concatenate Strings("MASTER ALARM (" ("string"), w525, ")" ("string")) -> (w526:string)
            n336 = Select(t=w526, s=w528, f="") -> (s? t:f=w527:string)
            n337 = Compound Arithmetic op=OR(w482, w481) -> (w480:bool)
            n338 = Select(t=cluster{u32, u32}[] [{6618880, 16448250}, {16448250, 16448250}] ("Colors [4]"), s=w473, f=cluster{u32, u32}[] [{16755474, 16448250}, {16448250, 16448250}] ("Colors [4]")) -> (s? t:f=w515:cluster{u32, u32}[])
            n339 = call "ReducedBWSendToNT.vim"("Value In"=w480, "NT Name"="Some_Switch_Armed" ("Name")) -> ()  [unwired: 1 out]
            n340 = property on="Master_Caution_GUI_0" class="Bool (strict)"("BoolText.Text"=w527) -> ()  [unwired: 2 in, 2 out]
            n341 = property on="Master_Caution_GUI_1" class="Bool (strict)"("BoolText.Text"=w527) -> ()  [unwired: 2 in, 2 out]
            n342 = property on="Master_Caution_GUI_2" class="Bool (strict)"("BoolText.Text"=w527) -> ()  [unwired: 2 in, 2 out]
            n343 = property on="Mute_Audible_Warnings" class="Bool"("Colors [4]"=w515) -> ()  [unwired: 2 in, 2 out]
            "WA_Ret_Left" <- FALSE ("WA_Ret_Left")
            "WA_Ret_Right" <- FALSE ("WA_Ret_Right")
            "LL_Ret_Left" <- FALSE ("LL_Ret_Left")
            "LL_Ret_Right" <- FALSE ("LL_Ret_Right")
          }
          frame #8 {
            # "Actuator Controls"
            n344 = Build Array("Motor 1 Amplitude", "Motor 2 Amplitude", "Motor 3 Amplitude", "Motor 4 Amplitude", "Motor 5 Amplitude", "Motor 6 Amplitude", "Motor 7 Amplitude", "Motor 8 Amplitude") -> (w543:dbl[])
            n345 = Build Array("Solenoid 1 Toggle", "Solenoid 2 Toggle", "Solenoid 3 Toggle", "Solenoid 4 Toggle") -> (w539:bool[])
            n346 = call "ReducedBWSendToNT.vim"("Value In"=w543, "NT Name"="Motor_Amplitudes") -> ()  [unwired: 1 out]
            n347 = call "ReducedBWSendToNT.vim"("Value In"=w539, "NT Name"="Solenoid_Toggles") -> ()  [unwired: 1 out]
            n348 = Build Array("Solenoid 1 Selector", "Solenoid 2 Selector", "Solenoid 3 Selector", "Solenoid 4 Selector") -> (w537:T23)
            n349 = Build Array("Motor 1 Button Selector", "Motor 2 Button Selector", "Motor 3 Button Selector", "Motor 4 Button Selector", "Motor 5 Button Selector", "Motor 6 Button Selector", "Motor 7 Button Selector", "Motor 8 Button Selector") -> (w540:T24)
            n350 = call "ReducedBWSendToNT.vim"("Value In"=w537, "NT Name"="Solenoid_Selector_States") -> ()  [unwired: 1 out]
            n351 = call "ReducedBWSendToNT.vim"("Value In"=w540, "NT Name"="Motor_Selector_States") -> ()  [unwired: 1 out]
          }
          frame #9 {
            # "flush NT tables"
            n352 = call <vilib>:"NT Flush Data Updates.vi"() -> ()  [unwired: 11 in, 1 out]
          }
        }
      }
    }
  }
  n353 = while {
    stop <- FALSE stop-if-true
    # "Set window properties"
    n354 = Not(x="Dock_Dashboard") -> (.not. x?=w569:bool)
    n355 = First Call?() -> (First Call?: T/F=w573:bool)
    n356 = Wait (ms)(milliseconds to wait=u32 10) -> ()  [unwired: 1 out]
    n357 = Compound Arithmetic op=OR(w569, w573) -> (w571:bool)
    n358 = control-ref of="This VI"() -> (w572:refnum<vi>)
    n359 = call "EdgeTrigger.vi"("Input Signal"=w571) -> ("Falling Edge Trigger"=w570:bool)  [unwired: 2 out]
    n360 = case shown="False" w571 {
      tunnel: w572 -> [w578 w585]
      tunnel: w570 -> [w576 _]
      frame False {
        n361 = case shown="True" w576 {
          tunnel: T25 {"Left"=100, "Top"=100, "Right"=1390, "Bottom"=585} ("Front Panel Window:Window Bounds") -> [_ w584]
          tunnel: w578 -> [w581 w583]
          tunnel: [w581 w582] -> w577
          frame False {
          }
          frame True {
            n362 = property class="VI"(reference=w583, "Front Panel.WinBounds"=w584) -> (reference out=w582:refnum<vi>)  [unwired: 1 in, 1 out]
          }
        }
        n363 = property class="VI"(reference=w577, "Front Panel.TitleBarVis"=TRUE ("Front Panel Window:Title Bar Visible")) -> ()  [unwired: 1 in, 2 out]
      }
      frame True {
        n364 = property class="VI"(reference=w585, "Front Panel.WinBounds"=T25 {"Left"=0, "Top"=0, "Right"=1290, "Bottom"=485} ("Front Panel Window:Window Bounds"), "Front Panel.TitleBarVis"=FALSE ("Front Panel Window:Title Bar Visible")) -> ()  [unwired: 1 in, 2 out]
      }
    }
  }
  n365 = while {
    tunnel: w20 -> [w591]
    tunnel: w19 -> [_]
    tunnel: w17 -> [w590]
    tunnel: w12 -> [w589]
    tunnel: w2 -> [w588]
    stop <- FALSE stop-if-true
    # "Process UI events related to test mode, checklist, and camera settings"
    n366 = event shown="[0] Timeout" {
      selector: w591 -> [_ _ _ _]
      dyn-events: _ -> [_ _ _ _]
      timeout: u32 60 ("milliseconds to wait") -> [_ _ _ _]
      tunnel: w590 -> [_ _ _ _]
      tunnel: w589 -> [_ _ _ _]
      tunnel: w588 -> [w594 _ _ _]
      event Timeout {
        (unwired) T1."Variables" ("Dashboard Tab")
        n367 = event-data() -> ()  [unwired: 1 in, 1 out]
        n368 = case shown="\"Variables\"" "Dashboard Tab" {
          tunnel: w594 -> [_ _ _]
          frame "Tune" {
          }
          frame "TeleOp", Default {
          }
          frame "Variables" {
            w599 = string[] ["CameraPublisher", "Usage", "DB"]  # Items to initially close
            n369 = First Call?() -> (First Call?: T/F=w600:bool)
            n370 = control-ref of="Tree"() -> (w601:refnum<vi>)
            n371 = Select(t=w599, s=w600, f=string[] []) -> (s? t:f=w597:string[])
            n372 = call <vilib>:"NT Read and Format Entries as Tree.vi"("Tags to  Close"=w597, "Tree Refnum"=w601) -> ()  [unwired: 8 in, 2 out]
          }
        }
        n373 = call <vilib>:"Connextion Info.vi"() -> ("Connected"=→"NT Connection":bool)  [unwired: 10 in, 1 out]
      }
      event "CheckList": Double Click {
        # "Shift clears all"
        # "Update symbols on the listbox"
        n374 = event-data() -> ("PlatMods.Shift"=w602:bool, "Row"=w604:i32)  [unwired: 1 in]
        n375 = case shown="True" w602 {
          tunnel: w604 -> [w608 _]
          tunnel: 1 -> [w607 _]
          frame False {
            n376 = property on="CheckList" class="LstBox (strict)"() -> ("Item Symbols"=w606:i32[])  [unwired: 2 in, 2 out]
            n377 = Replace Array Subset(array=w606, new element=w607, index=w608) -> (w605:i32[])
            n378 = property on="CheckList" class="LstBox (strict)"("Item Symbols"=w605) -> ()  [unwired: 2 in, 2 out]
          }
          frame True {
            w609 = 0 ("Top Row")
            n379 = property on="CheckList" class="LstBox (strict)"() -> ("Number of Rows"=w611:u32)  [unwired: 2 in, 2 out]
            n380 = Initialize Array(0, w611) -> (w610:i32[])
            n381 = property on="CheckList" class="LstBox (strict)"("Top Row"=w609, "Value"=w609, "Item Symbols"=w610) -> ()  [unwired: 2 in, 2 out]
          }
        }
      }
      event "CheckList": Key Down {
        # "Update symbols on the listbox\nLeft and right keys check and uncheck"
        n382 = event-data() -> ("VKey"=w614:T26)  [unwired: 1 in]
        n383 = case shown="\"Left\", \"Right\"" w614 {
          selector: w614 -> [w619 _]
          tunnel: eventvkey."Left" ("VKey") -> [w617 _]
          frame "Left", "Right" {
            n384 = Equal?(x=w617, y=w619) -> (x = y?=w618:bool)
            n385 = Select(t=0, s=w618, f=1) -> (s? t:f=w620:i32)
            n386 = property on="CheckList" class="LstBox (strict)"() -> ("Item Symbols"=w623:i32[])  [unwired: 2 in, 2 out]
            n387 = Replace Array Subset(array=w623, new element=w620, index="CheckList") -> (w622:i32[])
            n388 = property on="CheckList" class="LstBox (strict)"("Item Symbols"=w622) -> ()  [unwired: 2 in, 2 out]
          }
          frame Default {
          }
        }
      }
      event "Tree": Double Click {
        n389 = event-data() -> ("PlatMods"=w629:T27, "Tag"=w626:string)  [unwired: 1 in]
        n390 = Unbundle(w629) -> ("Shift"=w628:bool)  [unwired: 4 out]
        n391 = String Subset(string=w626, length (rest)=1 ("length (rest)")) -> (substring=w625:string)  [unwired: 1 in]
        n392 = Not(x=w628) -> (.not. x?=w627:bool)
        n393 = case shown="\"/\"" w625 {
          tunnel: w626 -> [_ w631]
          tunnel: w627 -> [_ w630]
          frame Default {
          }
          frame "/" {
            n394 = call <vilib>:"NT Update Persistence.vi"("Persistence"=w630, "Name"=w631) -> ()  [unwired: 9 in, 1 out]
          }
        }
      }
    }
  }
  n395 = while {
    tunnel: w3 -> [_]
    stop <- FALSE stop-if-true
    # "Maintain LimeLight connection"
    n396 = local read "Enable_Streaming_GUI"() -> (w632:bool)
    n397 = Wait (ms)(milliseconds to wait=u32 1000) -> ()  [unwired: 1 out]
    n398 = case shown="True" w632 {
      frame False {
      }
      frame True {
        w645 = "320x240 MJPEG 22 fps" ("String")
        w639 = "mjpg:http://10.42.65.11:5800"
        w644 = "/CameraPublisher/limelight/"
        # "manually configure the NT for a single LimeLight\ncamera in order to bypass WPILib's camera\nauto-detection which fails when the NTs are refreshed\nafter the code restarts on the roboRIO"
        n399 = Concatenate Strings("ip:http://", "10.42.65.11:5800" ("string")) -> (w647:string)
        n400 = Build Array(w639, w639) -> (w649:string[])
        n401 = Concatenate Strings(w644, "source") -> (w646:string)
        n402 = Concatenate Strings(w644, "description") -> (w650:string)
        n403 = Concatenate Strings(w644, "mode") -> (w651:string)
        n404 = Build Array(w645) -> (w653:string[])
        n405 = Concatenate Strings(w644, "streams") -> (w648:string)
        n406 = Concatenate Strings(w644, "modes") -> (w652:string)
        n407 = call-poly <vilib>:"NT Write Value.vi"("value"=w647, "name"=w646) -> ()  [unwired: 9 in, 1 out]
        n408 = call-poly <vilib>:"NT Write Value.vi"("value"="limelight" ("String"), "name"=w650) -> ()  [unwired: 9 in, 1 out]
        n409 = call-poly <vilib>:"NT Write Value.vi"("value"=w645, "name"=w651) -> ()  [unwired: 9 in, 1 out]
        n410 = call-poly <vilib>:"NT Write Value.vi"("value"=w649, "name"=w648) -> ()  [unwired: 9 in, 1 out]
        n411 = call-poly <vilib>:"NT Write Value.vi"("value"=w653, "name"=w652) -> ()  [unwired: 9 in, 1 out]
      }
    }
  }
  n412 = while {
    tunnel: u16 1741 ("timeout ms (25000)") -> [w655]
    stop <- FALSE stop-if-true
    # "Wait for DS connections"
    n413 = TCP Create Listener(10:w655) -> (0:w654:errorcluster, 3:w656:refnum<k5>)  [unwired: 4 in, 1 out]
    n414 = case shown="No Error" w654 {
      selector: w654 -> [w658 _]
      tunnel: w656 -> [w659 _]
      frame No Error {
        n415 = while {
          tunnel: w659 -> [w662]
          tunnel: w658 -> [w661]
          stop <- FALSE stop-if-true
          n416 = TCP Wait On Listener(8:w661, 11:w662) -> (0:w663:errorcluster, 4:w664:refnum<k5>)  [unwired: 2 in, 3 out]
          n417 = local write "TCP"(w664) -> ()
          n418 = case shown="Error" w663 {
            frame No Error {
            }
            frame Error {
              n419 = Wait (ms)(milliseconds to wait=u32 1000) -> ()  [unwired: 1 out]
            }
          }
        }
      }
      frame Error {
        n420 = Wait (ms)(milliseconds to wait=u32 1000) -> ()  [unwired: 1 out]
      }
    }
  }
  n421 = while {
    shift-right: [w677] -> _
    shift-left: _ -> [w730]
    shift-right: [w678] -> _
    shift-left: _ -> [w720]
    tunnel: w1 -> [_]
    stop <- FALSE stop-if-true
    # "Dynamic Overlays"
    n422 = To Long Integer(number="Reticule") -> (32bit integer=w711:i32)
    n423 = Wait (ms)(milliseconds to wait=u32 100) -> ()  [unwired: 1 out]
    n424 = Multiply(x=w711, y=2) -> (x*y=w710:i32)
    n425 = control-ref of="WA_Ret_Left"() -> (w691:refnum<vi>)
    n426 = control-ref of="WA_Ret_Right"() -> (w690:refnum<vi>)
    n427 = control-ref of="LL_Ret_Left"() -> (w676:refnum<vi>)
    n428 = control-ref of="LL_Ret_Right"() -> (w675:refnum<vi>)
    n429 = Increment(x=w710) -> (x+1=w697:i32)
    n430 = First Call?() -> (First Call?: T/F=w700:bool)
    n431 = Index Array(array=w720, index #1=w710, index #2=w697) -> (element #1=w714:i32, element #2=w722:i32)
    n432 = Or(x="Up", y="Down") -> (x .or. y?=w726:bool)
    n433 = Or(x="Left", y="Right") -> (x .or. y?=w716:bool)
    n434 = case shown="True" w700 {
      tunnel: [w741 w754] -> w677
      tunnel: w730 -> [w741 _]
      tunnel: w691 -> [_ w753]
      tunnel: w690 -> [_ w752]
      tunnel: w676 -> [_ w743]
      tunnel: w675 -> [_ w742]
      frame False {
      }
      frame True {
        n435 = property class="Bool (strict)"(reference=w753) -> ("Left"=w751:i32, "Top"=w750:i32)  [unwired: 1 in, 2 out]
        n436 = property class="Bool (strict)"(reference=w752) -> ("Left"=w749:i32, "Top"=w748:i32)  [unwired: 1 in, 2 out]
        n437 = property class="Bool (strict)"(reference=w743) -> ("Left"=w747:i32, "Top"=w746:i32)  [unwired: 1 in, 2 out]
        n438 = property class="Bool (strict)"(reference=w742) -> ("Left"=w745:i32, "Top"=w744:i32)  [unwired: 1 in, 2 out]
        n439 = Build Array(w751, w750, w749, w748, w747, w746, w745, w744) -> (w754:i32[])
      }
    }
    n440 = Bundle("WA_Ret_Left"=w691, "WA_Ret_Right"=w690, "LL_Ret_Left"=w676, "LL_Ret_Right"=w675) -> (w682:T28)  [unwired: 1 in]
    n441 = Decrement(x=w722) -> (x-1=w729:i32)
    n442 = Increment(x=w722) -> (x+1=w728:i32)
    n443 = Decrement(x=w714) -> (x-1=w719:i32)
    n444 = Increment(x=w714) -> (x+1=w718:i32)
    n445 = Select(t=w729, s="Up", f=w728) -> (s? t:f=w727:i32)
    n446 = Select(t=w719, s="Left", f=w718) -> (s? t:f=w717:i32)
    n447 = Select(t=w727, s=w726, f=w722) -> (s? t:f=w696:i32)
    n448 = Select(t=w717, s=w716, f=w714) -> (s? t:f=w715:i32)
    n449 = Replace Array Subset(array=w720, new element #1=w715, index #1=w710, new element #2=w696, index #2=w697) -> (w695:i32[])
    n450 = Current VI's Path() -> (path=w706:path)
    n451 = Strip Path(path=w706) -> (stripped path=w705:path)  [unwired: 1 out]
    n452 = Cluster To Array(cluster=w682) -> (array=w694:refnum<vi>[])
    n453 = Strip Path(path=w705) -> (stripped path=w704:path)  [unwired: 1 out]
    n454 = Array Size(array=w694) -> (size(s)=w693:i32)
    n455 = Build Path(base path=w704, name or relative path=path "reticule positions" ("XML File Path")) -> (appended path=w703:path)
    n456 = Multiply(x=2 ("dimension size"), y=w693) -> (x*y=w699:i32)
    n457 = Initialize Array(0, w699) -> (w689:i32[])
    n458 = call-poly <vilib>:"Read From XML File.vi"("XML File Path"=w703) -> ("error out"=w681:errorcluster, "XML Elements"=w702:string[])  [unwired: 8 in, 1 out]
    n459 = case shown="No Error" w681 {
      tunnel: w702 -> [w737 _]
      tunnel: w689 -> [w734 _]
      tunnel: [w733 i32[] [0, 0, 0, 0, 0, 0, 0, 0, 0, 0, 0, 0] ("value")] -> w679
      frame No Error {
        n460 = Index Array(array=w737, index=0) -> (element=w735:string)
        n461 = Unflatten From XML(xml string=w735, type=w734) -> (value=w733:i32[])  [unwired: 1 in, 1 out]
      }
      frame Error {
      }
    }
    n462 = First Call?() -> (First Call?: T/F=w721:bool)
    n463 = Select(t=w679, s=w721, f=w695) -> (s? t:f=w678:i32[])
    n464 = Add(x=w678, y=w677) -> (x+y=w680:i32[])
    n465 = Index Array(array=w680, index #1=0 ("index")) -> (element #1=w686:i32, element #2=w685:i32, element #3=w684:i32, element #4=w683:i32, element #5=w674:i32, element #6=w673:i32, element #7=w672:i32, element #8=w671:i32)  [unwired: 7 in]
    n466 = Unbundle(w682) -> ("WA_Ret_Left"=w687:refnum<vi>, "WA_Ret_Right"=w688:refnum<vi>, "LL_Ret_Left"=w670:refnum<vi>, "LL_Ret_Right"=w669:refnum<vi>)
    n467 = Flatten To XML(6:w678) -> (2:w708:string)
    n468 = call "EdgeTrigger.vi"("Input Signal"="Save") -> ("Rising Edge Trigger"=w667:bool)  [unwired: 2 out]
    n469 = case shown="True" w667 {
      tunnel: w708 -> [_ w740]
      tunnel: w703 -> [_ w739]
      frame False {
      }
      frame True {
        n470 = call-poly <vilib>:"Write to XML File.vi"("XML Input"=w740, "XML File Path"=w739) -> ()  [unwired: 7 in, 3 out]
      }
    }
    n471 = property class="Bool (strict)"(reference=w687, "Left"=w686, "Top"=w685) -> ()  [unwired: 1 in, 2 out]
    n472 = property class="Bool (strict)"(reference=w688, "Left"=w684, "Top"=w683) -> ()  [unwired: 1 in, 2 out]
    n473 = property class="Bool (strict)"(reference=w670, "Left"=w674, "Top"=w673) -> ()  [unwired: 1 in, 2 out]
    n474 = property class="Bool (strict)"(reference=w669, "Left"=w672, "Top"=w671) -> ()  [unwired: 1 in, 2 out]
  }
  n475 = while {
    tunnel: w10 -> [w784]
    tunnel: w3 -> [w768]
    tunnel: w4 -> [w766]
    stop <- FALSE stop-if-true
    w755 = u16 0 items=["Stop", "Record", "Playback Panel"] ("Rec Mode")
    # "Camera Feeds"
    n476 = First Call?() -> (First Call?: T/F=w762:bool)
    n477 = local read "NT Connection"() -> (w765:bool)
    n478 = call "Timer.vi"("Reset Timer"=w762) -> ("Time (ms)"=w761:u32)
    n479 = Greater?(x=w761, y=u32 5000) -> (0:w759:bool)
    n480 = Compound Arithmetic op=AND(w765, "Enable_Streaming_GUI", w759) -> (w764:bool)
    n481 = Bundle("Camera Name"="Camera Name", w768, "Saved DB Images Info"=w784) -> (w783:T29)  [unwired: 1 in]
    n482 = control-ref of="Camera Perf"() -> (w781:refnum<vi>)
    n483 = call <vilib>:"WPI_CameraRead MJPG for Dashboard_2.vi"("Camera Settings"="Camera Settings", "Rec Mode"=w755, "NT Connection"=w764, "Capture Info"=w783, "Image in"=w766) -> ("perf info"=w782:cluster{"Bandwidth (Mbps)":dbl, "fps":dbl}, "Active"=w767:bool, "Image\\ out"=w785:T3)  [unwired: 4 in]
    n484 = call <vilib>:"WPI_DashboardFormatPerf.vi"("Right Camera Perf"=cluster{"Bandwidth (Mbps)":dbl, "FPS":dbl} {"Bandwidth (Mbps)"=0.0, "FPS"=0.0}, "Performance"=w782, "String in"=w781) -> ()  [unwired: 9 in]
    n485 = case shown="True" w767 {
      tunnel: w785 -> [w796 w799]
      tunnel: [w796 w798] -> w780
      frame False {
        n486 = Wait Until Next ms Multiple(millisecond multiple=u32 500) -> ()  [unwired: 1 out]
      }
      frame True {
        # "image annotation etc."
        n487 = call "IMAQ Clear Overlay"("Image"=w799) -> ("Image Out"=w798:T3)  [unwired: 2 in, 8 out]
      }
    }
    n488 = call "IMAQ Rotate"("Angle (degrees)"=sgl 0.0, "Image Src"=w780) -> ("Image Dst Out"=w771:T3)  [unwired: 8 in, 1 out]
    n489 = call "IMAQ GetImageSize"("Image"=w771) -> ("Y Resolution"=w769:i32, "X Resolution"=w756:i32)  [unwired: 3 in, 1 out]
    n490 = To Double Precision Float(number=w756) -> (double precision float=w778:dbl)
    n491 = To Double Precision Float(number=w769) -> (double precision float=w777:dbl)
    n492 = Divide(x=w778, y=w777) -> (x/y=w776:dbl)
    n493 = Less?(x=w776, y=1.9) -> (x < y?=→"No_Secondary_Camera":bool)
    n494 = case shown="160, Default" w756 {
      tunnel: "Partial Video Stream" ("Image Name") -> [_ w795]
      tunnel: [w787 w794] -> w758
      tunnel: w771 -> [w787 w792]
      frame 320 {
        # "wide angle camera found"
      }
      frame 160, Default {
        w788 = T13 4 items=["Grayscale (U8)", "Grayscale (I16)", "Grayscale (SGL)", "Complex (CSG)", "RGB (U32)", "HSL (U32)", "RGB (U64)"] ("Image Type")
        # "no wide angle camera found"
        n495 = call "IMAQ Create"("Image Name"=w795, "Image Type"=w788) -> ("New Image"=w791:T3)  [unwired: 3 in, 1 out]
        n496 = call "IMAQ SetImageSize"("Y Resolution"=120, "X Resolution"=320, "Image"=w791) -> ("Image Out"=w793:T3)  [unwired: 2 in, 1 out]
        n497 = call "IMAQ ImageToImage 2"("Image Src (Small)"=w792, "Image Src (Large)"=w793) -> ("Image Dst Out"=w794:T3)  [unwired: 8 in, 1 out]
      }
    }
    "Combined Camera Feed" <- w758
  }
  n498 = while {
    stop <- FALSE stop-if-true
    # "Error Message Handling"
    n499 = property on="Actuator Testing" class="Ring (strict)"() -> ("RingText.Text"=w837:string)  [unwired: 2 in, 2 out]
    n500 = local read "Master_Safety_Override_1"() -> (w808:bool)
    n501 = local read "Arm_Calibrate_Wheels_GUI"() -> (w857:bool)
    n502 = local read "Arm_Calibrate_Joysticks"() -> (w827:bool)
    n503 = local read "Swerve_Shifter_Failure"() -> (w818:bool)
    n504 = local read "CAN_Bus_Fault_GUI"() -> (w824:bool)
    n505 = Wait (ms)(milliseconds to wait=u32 200) -> ()  [unwired: 1 out]
    n506 = local read "Swerve_Azimuth_Fault"() -> (w861:bool)
    n507 = local read "Home_Wheels_GUI"() -> (w810:bool)
    n508 = Not Equal?(x=w837, y="No_Test") -> (x != y?=w844:bool)
    n509 = local read "Swerve_Overheating"() -> (w870:bool)
    n510 = local read "Super_Test_Mode_GUI"() -> (w878:bool)
    n511 = call <vilib>:"Space Constant.vi"() -> ("String"=w835:string)
    n512 = local read "Swerve_Drive_Fault"() -> (w801:bool)
    n513 = local read "Auto_Test_Mode_GUI"() -> (w849:bool)
    n514 = local read "IMU_Failure_GUI"() -> (w841:bool)
    n515 = local read "Electrical_Fault_GUI"() -> (w832:bool)
    n516 = local read "Vision_Fault_GUI"() -> (w805:bool)
    n517 = local read "Pressure_Vent_GUI"() -> (w866:bool)
    n518 = local read "Auto_Error_GUI"() -> (w854:bool)
    n519 = Search and Replace String(replace all?=TRUE ("replace all? (F)"), input string=w837, search string="_", replace string=w835) -> (result string=w838:string)  [unwired: 4 in, 3 out]
    n520 = local read "Slow_Loop"() -> (w873:bool)
    n521 = Concatenate Strings("testing " ("string"), w838) -> (w847:string)
    n522 = Bundle("homing the wheels", "Home_Wheels_GUI"=w810, 60.0) -> (w809:cluster{string, "Home_Wheels_GUI":bool, dbl})  [unwired: 1 in]
    n523 = Bundle("swerve shifter failure, forced into low gear", "Swerve_Shifter_Failure"=w818, 600.0) -> (w817:T30)  [unwired: 1 in]
    n524 = Bundle("Lime Light failure", "Vision_Fault_GUI"=w805, 600.0) -> (w804:cluster{string, "Vision_Fault_GUI":bool, dbl})  [unwired: 1 in]
    n525 = Bundle("swerve drive failure", "Swerve_Drive_Fault"=w801, 600.0) -> (w800:cluster{string, "Swerve_Drive_Fault":bool, dbl})  [unwired: 1 in]
    n526 = Bundle("safeties disengaged", "Master_Safety_Override_1"=w808, 10.0) -> (w882:T31)  [unwired: 1 in]
    n527 = Bundle("disabled test mode", "Super_Test_Mode_GUI"=w878, 10.0) -> (w881:cluster{string, "Super_Test_Mode_GUI":bool, dbl})  [unwired: 1 in]
    n528 = Bundle("control latency too high", "Slow_Loop"=w873, 60.0) -> (w874:cluster{string, "Slow_Loop":bool, dbl})  [unwired: 1 in]
    n529 = Bundle("drive train overheating", "Swerve_Overheating"=w870, 60.0) -> (w869:cluster{string, "Swerve_Overheating":bool, dbl})  [unwired: 1 in]
    n530 = Bundle("pressure venting", "Pressure_Vent_GUI"=w866, 600.0) -> (w865:cluster{string, "Pressure_Vent_GUI":bool, dbl})  [unwired: 1 in]
    n531 = Bundle("swerve azimuth failure", "Swerve_Azimuth_Fault"=w861, 600.0) -> (w862:T32)  [unwired: 1 in]
    n532 = Bundle("ready to calibrate swerve modules", "Arm_Calibrate_Wheels_GUI"=w857, 10.0) -> (w858:T33)  [unwired: 1 in]
    n533 = Bundle("autonomous play failure", "Auto_Error_GUI"=w854, 10.0) -> (w853:cluster{string, "Auto_Error_GUI":bool, dbl})  [unwired: 1 in]
    n534 = Bundle("autonomous test mode", "Auto_Test_Mode_GUI"=w849, 10.0) -> (w850:cluster{string, "Auto_Test_Mode_GUI":bool, dbl})  [unwired: 1 in]
    n535 = Bundle(w847, w844, 10.0) -> (w843:cluster{string, bool, dbl})  [unwired: 1 in]
    n536 = Bundle("IMU failure, auto-targeting disabled", "IMU_Failure_GUI"=w841, 600.0) -> (w839:cluster{string, "IMU_Failure_GUI":bool, dbl})  [unwired: 1 in]
    n537 = Bundle("electrical bus fault, power down", "Electrical_Fault_GUI"=w832, 60.0) -> (w831:T34)  [unwired: 1 in]
    n538 = Bundle("ready to calibrate joysticks, wait ten seconds after pressing calibrate", "Arm_Calibrate_Joysticks"=w827, 10.0) -> (w828:T35)  [unwired: 1 in]
    n539 = Bundle("CAN bus fault, check wiring", "CAN_Bus_Fault_GUI"=w824, 60.0) -> (w826:cluster{string, "CAN_Bus_Fault_GUI":bool, dbl})  [unwired: 1 in]
    n540 = local read "Audible_Warnings_Enabled_GUI"() -> (w816:bool)
    n541 = Build Array(w882, w881, w874, w869, w865, w862, w858, w853, w850, w843, w839, w831, w828, w826, w817, w809, w804, w800) -> (w880:T36)
    n542 = call "EdgeTrigger.vi"("Input Signal"=w816) -> ("All Edge Trigger"=w815:bool)  [unwired: 2 out]
    n543 = call "ErrorMessageBuilder.vi"("Errors"=w880, "Reset Error History"=w815) -> ("Combined Error String"=w821:string)
    n544 = Not Equal?(x="", y=w821) -> (x != y?=w822:bool)
    n545 = Compound Arithmetic op=AND(w816, w822) -> (w814:bool)
    n546 = case shown="True" w814 {
      tunnel: w821 -> [_ w889]
      frame False {
      }
      frame True {
        n547 = call "TextToSpeech.vi"("Text To Be Spoken"=w889) -> ()  [unwired: 9 in, 2 out]
      }
    }
    n548 = case shown="True" w822 {
      tunnel: w821 -> [_ w888]
      frame False {
      }
      frame True {
        "Combined Error String" <- w888
      }
    }
  }
